vi "imp_test_v8_1.vi"() -> ()   [LabVIEW 2014]
uses:
  <vilib>/LabVIEW Targets/FPGA/cRIO/shared/nicrio_ModuleControls/nicrio_cRIO-9237_DataRatesRing.ctl
  <vilib>/LabVIEW Targets/FPGA/cRIO/shared/nicrio_ModuleControls/nicrio_cRIO-9237_ExcitationVoltageRing.ctl
  <vilib>/rvi/FXPMathLib/FxpSinAndCos/subVIs/nifxpmath_SinAndCos_SimConfig.ctl
  <vilib>/rvi/Emulation/niFpgaGetClockAttributes.vi
  <vilib>/rvi/Emulation/niFpgaSctlEmulationGetInTimedLoop.vi
  <vilib>/rvi/Emulation/niFpgaEmulationReportErrorSimple.vi
  <vilib>/rvi/Emulation/niFpgaProcessEmulError.vi
  <vilib>/rvi/interface/RandomDataEmulation/nirviRandomDataMultiElementFPGAFIFO.vi
  <instcachedir>/0/nirviRandomDataMultiElementFPGAFIFO_AD0CFC12EF974623A9C2E4184BC062B2.lvgen/nirviRandomDataMultiElementFPGAFIFO_AD0CFC12EF974623A9C2E4184BC062B2_025.vi
  <vilib>/rvi/interface/RandomDataEmulation/niFpgaRandomDataHandleErrors.vi
  <vilib>/rvi/Emulation/niFpgaCriticalErrorInLSC.vi
  <vilib>/rvi/FXPMathLib/FxpSinAndCos/simVIs/DllFxpSinAndCosTemp_sub.vi
  <vilib>/rvi/eio/common/nirviEmuTemplateMethod_errors.vi
  <vilib>/rvi/eio/common/nirviEmuTemplatePropertySet_errors.vi
  <vilib>/rvi/DataTransferAndStorage/Container/XNode/niFpgaContainer.xnode
  <vilib>/rvi/interface/RandomDataEmulation/nirviRandomDataFpgaMultiElementTemplate.vi
  <vilib>/rvi/FXPMathLib/FxpSinAndCos/XNode/nifxpmath_SinAndCos.xnode
  <vilib>/eio/EIONode/EIONode.xnode
  <vilib>/rvi/Analysis/measure/butterworth/XNode/niFpgaButterworthFilter.xnode
  <vilib>/eio/EIOPropertyNode/EIOPropertyNode.xnode
  <vilib>/rvi/eio/common/nirviEmuTemplatePropertyGet_errors.vi
  <vilib>/rvi/eio/common/nirviEmuTemplatePropertyGet_noerrors.vi
  <vilib>/rvi/eio/common/nirviEmuTemplatePropertySet_noerrors.vi
panel:
  out "Dy_d (Mavg w. f.)":fxp<+/-,36,14>
  out "Dp_d (Mavg w. f.)":fxp<+/-,36,14>
  in  "Dp_d (Mavg) coeff.":i32[](array[numeric])=[946630756, 63555534]
  in  "Dy_d (Mavg) coeff.":i32[](array[numeric])=[946630756, 63555534]
  out "omega_y (Mavg w. f.)":fxp<+/-,36,14>
  in  "omega_y(Mavg) coeff.":i32[](array[numeric])=[946630756, 63555534]
  out "omega_p (Mavg w. f)":fxp<+/-,36,14>
  in  "omega_P(Mavg) coeff.":i32[](array[numeric])=[946630756, 63555534]
  in  "FIFO":i16(ring) items=["Pitch_F+P", "imp ctrl", "Yaw_F+P"]
  out "PID (kHz)":fxp<+/-,20,10>
  in  "Set 6":bool
  in  "Set 5":bool
  in  "Set 4":bool
  in  "Set 3":bool
  in  "Set 2":bool
  in  "Set 1":bool
  out "Dy1_d (T)":fxp<+/-,36,13>
  out "omega_y1 (T)":fxp<+/-,36,13>
  out "Dp1_d (T)":fxp<+/-,36,13>
  out "omega_p1 (T)":fxp<+/-,36,13>
  out "Dy2_d (T)":fxp<+/-,36,13>
  out "Dp2_d (T)":fxp<+/-,36,13>
  out "omega_y2 (T)":fxp<+/-,36,13>
  out "omega_p2 (T)":fxp<+/-,36,13>
  out "mt_omega_y2":u32
  out "mt_omega_p2":u32
  out "rad_y2":fxp<+/-,33,20>
  out "D_y2":fxp<+/-,32,7>
  out "rad_y1":fxp<+/-,33,20>
  out "D_y1":fxp<+/-,32,7>
  out "Encoder Position_y1":i32
  out "Encoder Position_y2":i32
  out "Encoder Position_p2":i32
  out "D_p2":fxp<+/-,32,7>
  out "rad_p2":fxp<+/-,33,20>
  out "D_p1":fxp<+/-,32,7>
  out "rad_p1":fxp<+/-,33,20>
  out "Encoder Position_p1":i32
  in  "Mag. factor_y":fxp<+/-,20,3>
  in  "Mag. encoder_y":bool
  out "omega_y (rad/s)":fxp<+/-,36,13>
  out "Dy_d (mm/s)":fxp<+/-,36,13>
  in  "Vy. Est.":i16(ring) items=["T", "Mavg", "Mavg w. f."]
  out "omega_y (Mavg)":fxp<+/-,36,14>
  out "Dy_d (Mavg)":fxp<+/-,36,14>
  in  "Dy_d_M_avg_Tc (uSec)":i32
  out "Dp_d (Mavg)":fxp<+/-,36,14>
  out "omega_p (Mavg)":fxp<+/-,36,14>
  in  "Dp_d_M_avg_Tc (uSec)":i32
  out "Dp_d (T)":fxp<+/-,36,13>
  out "omega_p (T)":fxp<+/-,36,13>
  in  "Vp. Est.":i16(ring) items=["T", "Mavg", "Mavg w. f."]
  in  "Mag. factor_p":fxp<+/-,20,3>
  in  "Mag. encoder_p":bool
  in  "Belt_out_p":fxp<+/-,7,7>
  in  "Belt_in_p":fxp<+/-,6,6>
  in  "Belt_out_y":fxp<+/-,7,7>
  in  "Belt_in_y":fxp<+/-,6,6>
  out "Fp_dc":fxp<+/-,32,10>
  out "Fy_dc":fxp<+/-,32,10>
  in  "Zero_y":bool
  in  "Zero_p":bool
  in  "mt0_omega_p":u32
  in  "Encoder reset":bool
  out "fpt_d":fxp<+/-,36,18>
  out "Dp_error_dd":fxp<+/-,36,16>
  out "Dp_error_d":fxp<+/-,33,8>
  in  "Dp_dd coeff.":i32[](array[numeric])=[946630756, 63555534]
  out "Dp_dd":fxp<+/-,36,25>
  out "dFp_PID":fxp<+/-,36,18>
  in  "dFp_PID coeff.":i32[](array[numeric])=[946630756, 63555534]
  out "fpt_i":fxp<+/-,34,18>
  in  "Bv_p":fxp<+/-,22,8>
  in  "Kv_p":fxp<+/-,22,8>
  out "Dp_error":fxp<+/-,22,7>
  out "Dpr_sin":fxp<+/-,22,7>
  in  "Sin offset_p":fxp<+/-,22,7>
  in  "Sin magnitude_p":fxp<+/-,21,6>
  out "Dpr_sin_dd":fxp<+/-,35,20>
  out "Dpr_sin_d":fxp<+/-,33,15>
  out "Sin omega_p":fxp<+/-,34,9>
  in  "Sin wave freq._p (Hz)":fxp<+/-,32,6>
  in  "Dpr_step":fxp<+/-,22,7>
  out "Dpr_for":fxp<+/-,22,7>
  in  "Command_p":i16(ring) items=["Step", "Sine"]
  in  "Ki_p":fxp<+/-,30,9>
  out "Fp_PID":fxp<+/-,36,16>
  in  "fp_tolorance":fxp<+,22,6>
  out "fp_tilde":fxp<+/-,33,10>
  in  "Kd_p":fxp<+/-,30,9>
  in  "Kp_p":fxp<+/-,32,13>
  out "Fr_p":fxp<+/-,32,10>
  in  "S/F coeff_p":fxp<+/-,25,-10>
  in  "S/F coeff_y":fxp<+/-,25,-10>
  out "va_p":fxp<+/-,36,7>
  out "vb_p":fxp<+/-,37,8>
  out "vq_p_F":fxp<+/-,20,5> format="%.57g"
  out "vd_p_F":fxp<+/-,20,5>
  in  "dFp_add":bool
  in  "Stop motor_p":bool
  out "Force_p":fxp<+/-,32,10>
  in  "Strain selection_p":i16(ring) items=["Raw", "Avg.8", "Avg.8 w. filter"]
  out "Strain_p (Avg8 w. f)":fxp<+/-,36,8>
  in  "Strain_p Avg.8 coeff.":i32[](array[numeric])=[946630756, 63555534]
  out "Strain_p (Avg8)":fxp<+/-,36,4>
  out "Raw Strain_p":fxp<+/-,36,4>
  out "Mod6/AI3":fxp<+/-,36,4>
  in  "Strain gage reset_p":bool
  out "Dp_d (mm/s)":fxp<+/-,36,13>
  out "omega_p (rad/s)":fxp<+/-,36,13>
  out "mt_omega_p1":u32
  out "rad_p(NrTheta)":fxp<+/-,33,20>
  out "D_p(mm)":fxp<+/-,32,7>
  out "Encoder Position_p":i32
  in  "Encoder reset_p":bool
  out "Strain_y (Avg8 w. f)":fxp<+/-,36,8>
  in  "Strain_y Avg8 coeff.":i32[](array[numeric])=[-898916953, 1957103773, 3888751]
  out "Dyr_for":fxp<+/-,22,7>
  in  "Command_y":i16(ring) items=["Step", "Sine"]
  out "Strain_y (Avg8)":fxp<+/-,36,4>
  in  "Strain selection_y":i16(ring) items=["Raw", "Avg.8", "Avg.8 w. filter"]
  out "vb_y":fxp<+/-,38,8>
  out "va_y":fxp<+/-,38,8>
  out "fyt_d":fxp<+/-,36,18>
  out "Fr_y":fxp<+/-,32,10>
  in  "Bv_y":fxp<+/-,22,8>
  out "Dy_error_dd":fxp<+/-,36,16>
  out "Dy_error_d":fxp<+/-,33,8>
  in  "Kv_y":fxp<+/-,22,8>
  out "Dy_error":fxp<+/-,22,7>
  out "Dyr_sin_dd":fxp<+/-,35,20>
  out "Dyr_sin_d":fxp<+/-,33,15>
  out "Sin omega_y":fxp<+/-,34,9>
  out "Dyr_sin":fxp<+/-,22,7>
  in  "Sin offset_y":fxp<+/-,22,7>
  in  "Sin magnitude_y":fxp<+/-,21,6>
  out "Time now(s)":fxp<+,52,14>
  in  "Sin wave freq._y (Hz)":fxp<+/-,32,6>
  in  "Dyr_step":fxp<+/-,22,7>
  in  "Drive mode":i16(ring) items=["Backward", "Forward"]
  out "Dy_dd":fxp<+/-,36,25>
  in  "Dy_dd coeff.":i32[](array[numeric])=[946630756, 63555534]
  out "dFy_PID":fxp<+/-,36,18>
  in  "dFy_PID coeff.":i32[](array[numeric])=[946630756, 63555534]
  out "fyt_i":fxp<+/-,36,16>
  out "Fy_PID":fxp<+/-,36,16>
  in  "fy_tolorance":fxp<+,22,6>
  in  "Ki_y":fxp<+/-,30,9>
  in  "Kd_y":fxp<+/-,30,9>
  out "fy_tilde":fxp<+/-,32,10>
  in  "Kp_y":fxp<+/-,32,13>
  out "vq_y_F":fxp<+/-,20,5> format="%.57g"
  out "vd_y_F":fxp<+/-,20,5>
  in  "dFy_add":bool
  in  "Stop motor_y":bool
  out "Dy_d (T)":fxp<+/-,36,13>
  out "omega_y (T)":fxp<+/-,36,13>
  in  "mt0_omega_y":u32
  out "mt_omega_y1":u32
  out "rad_y(NrTheta)":fxp<+/-,33,20>
  out "D_y(mm)":fxp<+/-,32,7>
  out "Encoder Position_y":i32
  in  "Encoder reset_y":bool
  in  "Ini coe.":bool
  out "Loop rate (kHz)":fxp<+/-,36,7>
  out "Force_y":fxp<+/-,32,10>
  out "Raw Strain_y":fxp<+/-,36,4>
  in  "Strain gage reset_y":bool
  in  "Stop (Strain)":bool
  out "Mod6/AI2":fxp<+/-,36,4>
  in  "Excitation Voltage":T1 items=["2.5 Volts", "3.3 Volts", "5.0 Volts", "10.0 Volts", "External Excitation"]
  in  "Data Rate":T2=1 items=["50.000 kS/s (NI 9237)"=1, "25.000 kS/s (NI 9237)"=2, "16.667 kS/s (NI 9237)"=3, "12.500 kS/s (NI 9237)"=4, "10.000 kS/s (NI 9237)"=5, "8.333 kS/s (NI 9237)"=6, "7.143 kS/s (NI 9237)"=7, "6.250 kS/s (NI 9237)"=8, "5.556 kS/s (NI 9237)"=9, "5.000 kS/s (NI 9237)"=10, "4.545 kS/s (NI 9237)"=11, "4.167 kS/s (NI 9237)"=12, "3.846 kS/s (NI 9237)"=13, "3.571 kS/s (NI 9237)"=14, "3.333 kS/s (NI 9237)"=15, "3.125 kS/s (NI 9237)"=16, "2.941 kS/s (NI 9237)"=17, "2.778 kS/s (NI 9237)"=18, "2.632 kS/s (NI 9237)"=19, "2.500 kS/s (NI 9237)"=20, "2.381 kS/s (NI 9237)"=21, "2.273 kS/s (NI 9237)"=22, "2.174 kS/s (NI 9237)"=23, "2.083 kS/s (NI 9237)"=24, "2.000 kS/s (NI 9237)"=25, "1.923 kS/s (NI 9237)"=26, "1.852 kS/s (NI 9237)"=27, "1.786 kS/s (NI 9237)"=28, "1.724 kS/s (NI 9237)"=29, "1.667 kS/s (NI 9237)"=30, "1.613 kS/s (NI 9237)"=31]
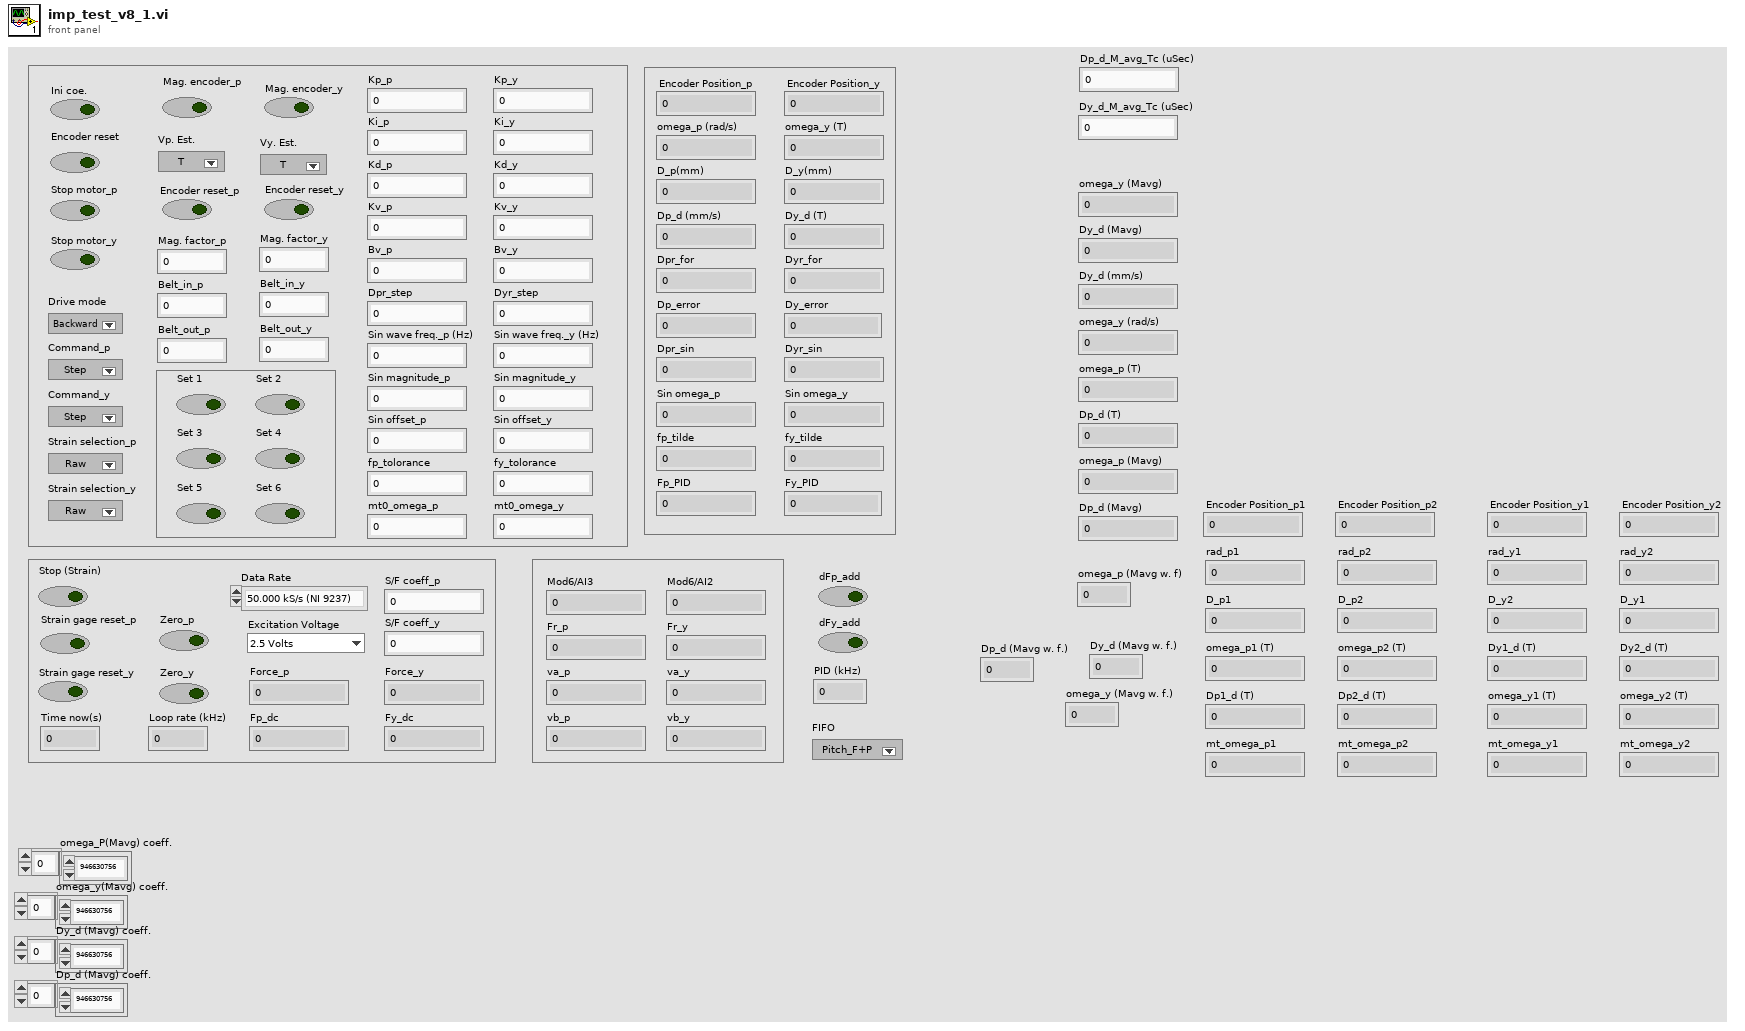
[diagram p1: front panel]
types:
  T1 = typedef "nicrio_cRIO-9237_ExcitationVoltageRing.ctl" = u8
  T2 = typedef "nicrio_cRIO-9237_DataRatesRing.ctl" = u8
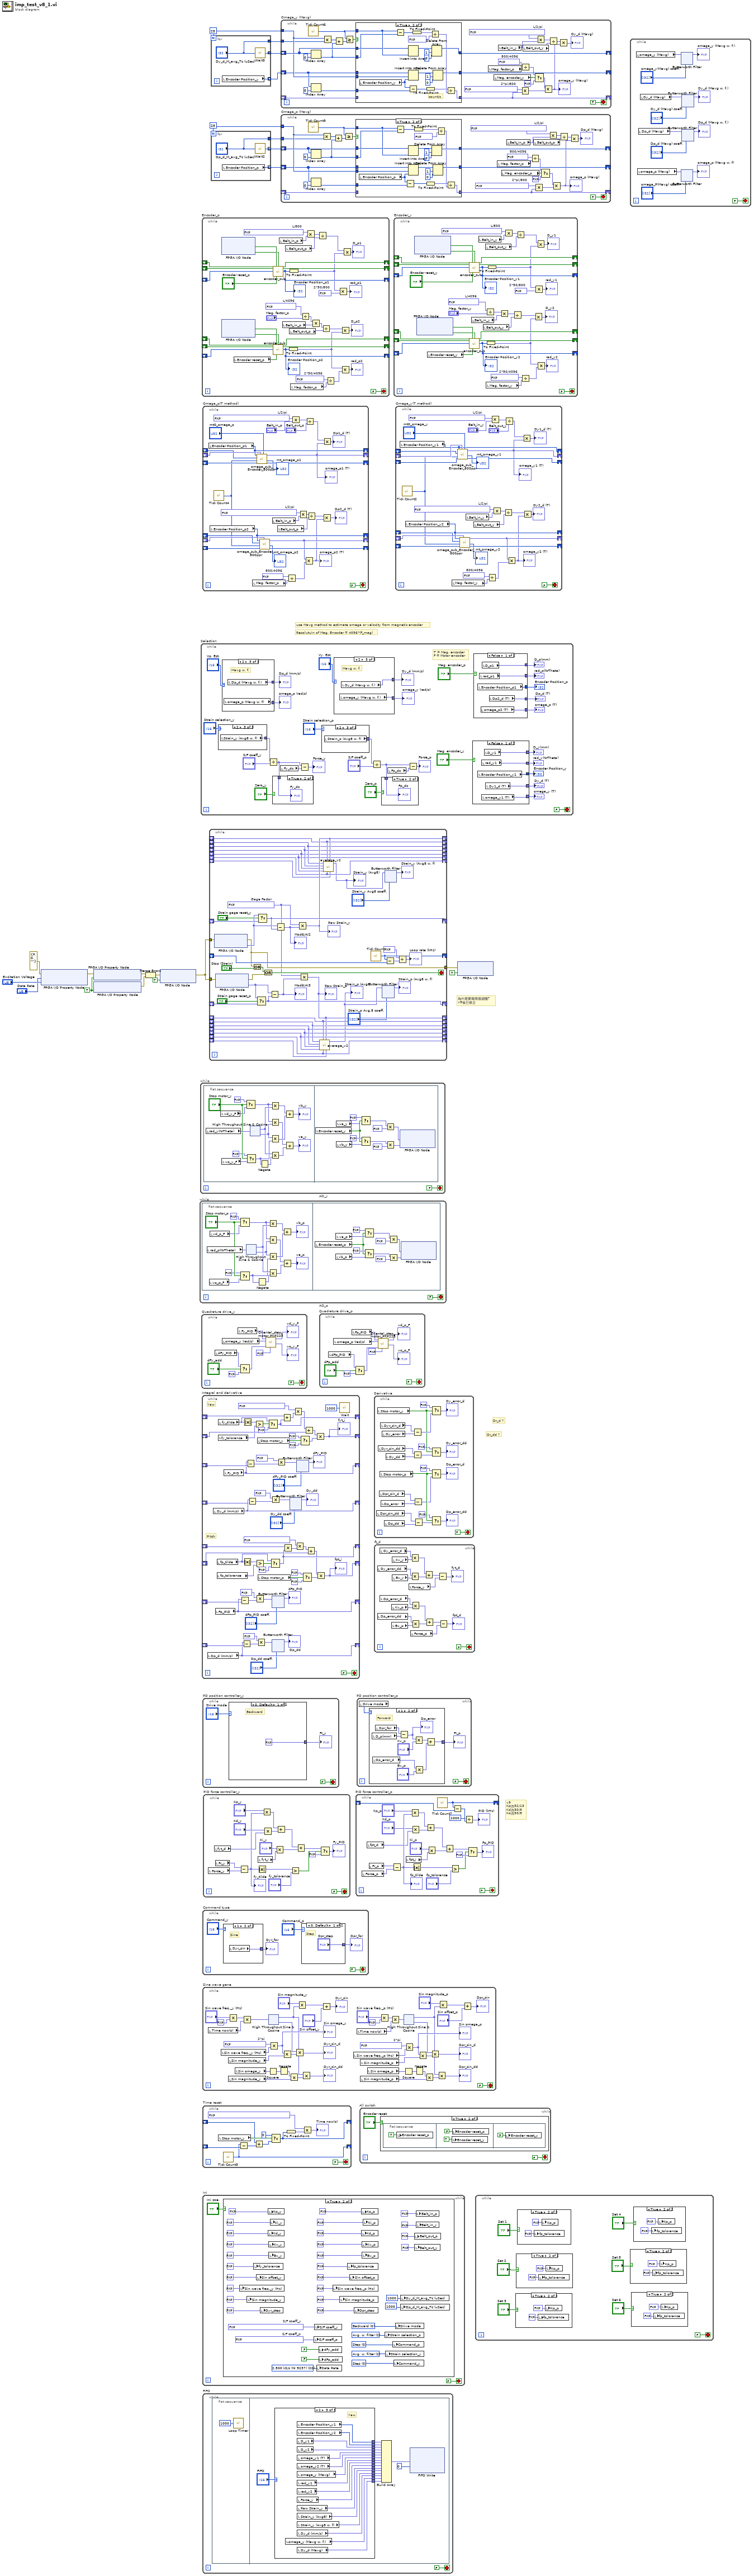
[diagram p0: block diagram]
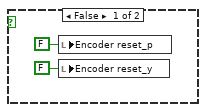
[diagram p10: hidden frame]
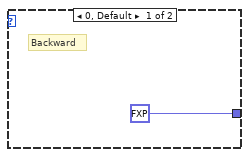
[diagram p11: hidden frame]
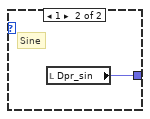
[diagram p12: hidden frame]
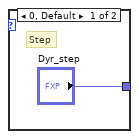
[diagram p13: hidden frame]
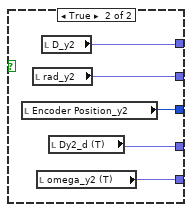
[diagram p14: hidden frame]
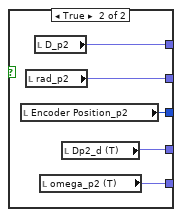
[diagram p15: hidden frame]
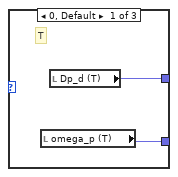
[diagram p16: hidden frame]
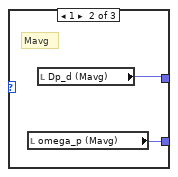
[diagram p17: hidden frame]
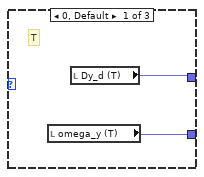
[diagram p18: hidden frame]
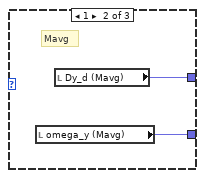
[diagram p19: hidden frame]
diagram:
  w5 = 25
  w8 = 25
  w13 = TRUE ("Half-Bridge Enable")
  # "v9\nKp改32/13\nKd改30/9\nKo改30/9"
  # "Resolutuin of Mag. Encoder = 4096*(F_mag)"
  # "use Mavg method to estimate omega or velocity from magnetic encoder"
  # "為什麼要寫兩個迴圈?\nv9後已修正"
  # "Dr_dd ?"
  # "Dr_d ?"
  n1 = xnode "FPGA I/O Property Node"("error in"=errorcluster {"status"=FALSE, "code"=0, "source"=""}, "Data Rate"="Data Rate", "Excitation Voltage"="Excitation Voltage") -> ("error out"=w18:errorcluster)  [unwired: 1 in, 1 out]
  n2 = xnode "FPGA I/O Property Node"("error in"=w18, "Half-Bridge Enable"=w13) -> ("error out"=w11:errorcluster)  [unwired: 1 in, 1 out]
  n3 = xnode "FPGA I/O Property Node"("Half-Bridge Enable"=w13) -> ("error out"=w10:errorcluster)  [unwired: 2 in, 1 out]
  n4 = Merge Errors(w11, w10) -> (w12:errorcluster)
  n5 = xnode "FPGA I/O Node"("error in"=w12, "Mod6/Start"=TRUE) -> ("error out"=w16:errorcluster)  [unwired: 1 in, 1 out]
  n6 = while "AO_p" {
    stop <- FALSE stop-if-true
    n7 = flat-sequence {
      frame #0 {
        n8 = local read "rad_p(NrTheta)"() -> (w33:fxp<+/-,33,20>)
        n9 = local read "vq_p_F"() -> (w34:fxp<+/-,20,5>)
        n10 = local read "vd_p_F"() -> (w36:fxp<+/-,20,5>)
        n11 = Select(t=fxp<+/-,20,5> 0.0, s="Stop motor_p", f=w36) -> (s? t:f=w25:fxp<+/-,20,5>)
        n12 = Select(t=fxp<+,1,1> 0.0, s="Stop motor_p", f=w34) -> (s? t:f=w24:fxp<+/-,20,5>)
        n13 = xnode "High Throughput Sine & Cosine"("x (pi)"=w33) -> ("sin(x)"=w27:fxp<+/-,16,2>, "cos(x)"=w26:fxp<+/-,16,2>)
        n14 = Negate(x=w24) -> (-x=w32:fxp<+/-,21,6>)
        n15 = Multiply(x=w25, y=w27) -> (x*y=w31:fxp<+/-,36,7>)
        n16 = Multiply(x=w25, y=w26) -> (x*y=w29:fxp<+/-,36,7>)
        n17 = Multiply(x=w26, y=w24) -> (x*y=w30:fxp<+/-,36,7>)
        n18 = Multiply(x=w27, y=w32) -> (x*y=w28:fxp<+/-,35,6>)
        n19 = Add(x=w31, y=w30) -> (x+y=→"vb_p":fxp<+/-,37,8>)
        n20 = Add(x=w29, y=w28) -> (x+y=→"va_p":fxp<+/-,36,7>)
      }
      frame #1 {
        n21 = local read "Encoder reset_p"() -> (w69:bool)
        n22 = local read "vb_p"() -> (w70:fxp<+/-,37,8>)
        n23 = local read "va_p"() -> (w71:fxp<+/-,36,7>)
        n24 = Select(t=fxp<+,2,2> 3.0, s=w69, f=w71) -> (s? t:f=w77:fxp<+/-,36,7>)
        n25 = Select(t=fxp<+,1,1> 0.0, s=w69, f=w70) -> (s? t:f=w76:fxp<+/-,37,8>)
        n26 = Multiply(x=w77, y=fxp<+/-,1,0> -0.5) -> (x*y=w72:fxp<+/-,36,6>)
        n27 = Multiply(x=w76, y=fxp<+/-,1,0> -0.5) -> (x*y=w73:fxp<+/-,36,6>)
        n28 = xnode "FPGA I/O Node"("Mod8/AO0"=w72, "Mod8/AO1"=w73) -> ()  [unwired: 2 in, 2 out]
      }
    }
  }
  n29 = while "AO_y" {
    stop <- FALSE stop-if-true
    n30 = flat-sequence {
      frame #0 {
        n31 = local read "rad_y(NrTheta)"() -> (w97:fxp<+/-,33,20>)
        n32 = local read "vd_y_F"() -> (w95:fxp<+/-,20,5>)
        n33 = local read "vq_y_F"() -> (w94:fxp<+/-,20,5>)
        n34 = Select(t=fxp<+/-,20,5> 0.0, s="Stop motor_y", f=w95) -> (s? t:f=w89:fxp<+/-,20,5>)
        n35 = Select(t=fxp<+/-,20,5> 0.0, s="Stop motor_y", f=w94) -> (s? t:f=w88:fxp<+/-,20,5>)
        n36 = xnode "High Throughput Sine & Cosine"("x (pi)"=w97) -> ("sin(x)"=w91:fxp<+/-,17,2>, "cos(x)"=w90:fxp<+/-,17,2>)
        n37 = Negate(x=w88) -> (-x=w87:fxp<+/-,21,6>)
        n38 = Multiply(x=w89, y=w91) -> (x*y=w86:fxp<+/-,37,7>)
        n39 = Multiply(x=w89, y=w90) -> (x*y=w84:fxp<+/-,37,7>)
        n40 = Multiply(x=w90, y=w88) -> (x*y=w85:fxp<+/-,37,7>)
        n41 = Multiply(x=w91, y=w87) -> (x*y=w83:fxp<+/-,36,6>)
        n42 = Add(x=w86, y=w85) -> (x+y=→"vb_y":fxp<+/-,38,8>)
        n43 = Add(x=w84, y=w83) -> (x+y=→"va_y":fxp<+/-,37,7>)
      }
      frame #1 {
        n44 = local read "Encoder reset_y"() -> (w130:bool)
        n45 = local read "va_y"() -> (w129:fxp<+/-,38,8>)
        n46 = local read "vb_y"() -> (w128:fxp<+/-,38,8>)
        n47 = Select(t=fxp<+,2,2> 3.0, s=w130, f=w129) -> (s? t:f=w134:fxp<+/-,38,8>)
        n48 = Select(t=fxp<+,1,1> 0.0, s=w130, f=w128) -> (s? t:f=w133:fxp<+/-,38,8>)
        n49 = Multiply(x=w134, y=fxp<+/-,1,0> -0.5) -> (x*y=w137:fxp<+/-,39,8>)
        n50 = Multiply(x=w133, y=fxp<+/-,1,0> -0.5) -> (x*y=w138:fxp<+/-,37,6>)
        n51 = xnode "FPGA I/O Node"("Mod8/AO2"=w137, "Mod8/AO3"=w138) -> ()  [unwired: 2 in, 2 out]
      }
    }
  }
  n52 = while "Selection" {
    stop <- FALSE stop-if-true
    # "T = Mag. encoder\nF = Motor encoder"
    n53 = case shown="2" "Strain selection_y" {
      tunnel: [w209 w210 w211] -> w170
      frame 0, Default {
        n54 = local read "Raw Strain_y"() -> (w209:fxp<+/-,36,4>)
      }
      frame 1 {
        n55 = local read "Strain_y (Avg8)"() -> (w210:fxp<+/-,36,4>)
      }
      frame 2 {
        n56 = local read "Strain_y (Avg8 w. f)"() -> (w211:fxp<+/-,36,8>)
      }
    }
    n57 = case shown="2" "Vp. Est." {
      tunnel: [w193 w194 w197] -> w153
      tunnel: [w192 w195 w196] -> w154
      frame 0, Default {
        # "T"
        n58 = local read "omega_p (T)"() -> (w193:fxp<+/-,36,13>)
        n59 = local read "Dp_d (T)"() -> (w192:fxp<+/-,36,13>)
      }
      frame 1 {
        # "Mavg"
        n60 = local read "omega_p (Mavg)"() -> (w194:fxp<+/-,36,14>)
        n61 = local read "Dp_d (Mavg)"() -> (w195:fxp<+/-,36,14>)
      }
      frame 2 {
        # "Mavg w. f."
        n62 = local read "omega_p (Mavg w. f)"() -> (w197:fxp<+/-,36,14>)
        n63 = local read "Dp_d (Mavg w. f.)"() -> (w196:fxp<+/-,36,14>)
      }
    }
    "Dp_d (mm/s)" <- w154
    "omega_p (rad/s)" <- w153
    n64 = Divide(x=w170, y="S/F coeff_y") -> (x/y=w163:fxp<+/-,32,10>)
    n65 = case shown="True" "Zero_y" {
      tunnel: w163 -> [_ w205]
      frame False {
      }
      frame True {
        "Fy_dc" <- w205
      }
    }
    n66 = local read "Fy_dc"() -> (w164:fxp<+/-,32,10>)
    n67 = Subtract(x=w163, y=w164) -> (x-y=→"Force_y":fxp<+/-,33,11>)
    n68 = case shown="2" "Strain selection_p" {
      tunnel: [w206 w207 w208] -> w168
      frame 0, Default {
        n69 = local read "Raw Strain_p"() -> (w206:fxp<+/-,36,4>)
      }
      frame 1 {
        n70 = local read "Strain_p (Avg8)"() -> (w207:fxp<+/-,36,4>)
      }
      frame 2 {
        n71 = local read "Strain_p (Avg8 w. f)"() -> (w208:fxp<+/-,36,8>)
      }
    }
    n72 = case shown="2" "Vy. Est." {
      tunnel: [w199 w201 w203] -> w156
      tunnel: [w198 w200 w202] -> w157
      frame 0, Default {
        # "T"
        n73 = local read "omega_y (T)"() -> (w198:fxp<+/-,36,13>)
        n74 = local read "Dy_d (T)"() -> (w199:fxp<+/-,36,13>)
      }
      frame 1 {
        # "Mavg"
        n75 = local read "omega_y (Mavg)"() -> (w200:fxp<+/-,36,14>)
        n76 = local read "Dy_d (Mavg)"() -> (w201:fxp<+/-,36,14>)
      }
      frame 2 {
        # "Mavg w. f."
        n77 = local read "omega_y (Mavg w. f.)"() -> (w202:fxp<+/-,36,14>)
        n78 = local read "Dy_d (Mavg w. f.)"() -> (w203:fxp<+/-,36,14>)
      }
    }
    "Dy_d (mm/s)" <- w156
    "omega_y (rad/s)" <- w157
    n79 = Divide(x=w168, y="S/F coeff_p") -> (x/y=w160:fxp<+/-,32,10>)
    n80 = case shown="True" "Zero_p" {
      tunnel: w160 -> [_ w204]
      frame False {
      }
      frame True {
        "Fp_dc" <- w204
      }
    }
    n81 = local read "Fp_dc"() -> (w158:fxp<+/-,32,10>)
    n82 = Subtract(x=w160, y=w158) -> (x-y=→"Force_p":fxp<+/-,33,11>)
    n83 = case shown="False" "Mag. encoder_y" {
      tunnel: [w176 w180] -> w144
      tunnel: [w175 w181] -> w145
      tunnel: [w174 w179] -> w147
      tunnel: [w172 w178] -> w141
      tunnel: [w173 w177] -> w140
      frame False {
        n84 = local read "Encoder Position_y1"() -> (w174:i32)
        n85 = local read "rad_y1"() -> (w176:fxp<+/-,33,20>)
        n86 = local read "omega_y1 (T)"() -> (w172:fxp<+/-,36,13>)
        n87 = local read "D_y1"() -> (w175:fxp<+/-,32,7>)
        n88 = local read "Dy1_d (T)"() -> (w173:fxp<+/-,36,13>)
      }
      frame True {
        n89 = local read "Encoder Position_y2"() -> (w179:i32)
        n90 = local read "rad_y2"() -> (w180:fxp<+/-,33,20>)
        n91 = local read "omega_y2 (T)"() -> (w178:fxp<+/-,36,13>)
        n92 = local read "D_y2"() -> (w181:fxp<+/-,32,7>)
        n93 = local read "Dy2_d (T)"() -> (w177:fxp<+/-,36,13>)
      }
    }
    "D_y(mm)" <- w145
    "rad_y(NrTheta)" <- w144
    "Encoder Position_y" <- w147
    "Dy_d (T)" <- w140
    "omega_y (T)" <- w141
    n94 = case shown="False" "Mag. encoder_p" {
      tunnel: [w186 w191] -> w149
      tunnel: [w185 w190] -> w150
      tunnel: [w184 w189] -> w151
      tunnel: [w182 w188] -> w143
      tunnel: [w183 w187] -> w142
      frame False {
        n95 = local read "Encoder Position_p1"() -> (w184:i32)
        n96 = local read "rad_p1"() -> (w185:fxp<+/-,33,20>)
        n97 = local read "omega_p2 (T)"() -> (w182:fxp<+/-,36,13>)
        n98 = local read "D_p1"() -> (w186:fxp<+/-,32,7>)
        n99 = local read "Dp2_d (T)"() -> (w183:fxp<+/-,36,13>)
      }
      frame True {
        n100 = local read "Encoder Position_p2"() -> (w189:i32)
        n101 = local read "rad_p2"() -> (w190:fxp<+/-,33,20>)
        n102 = local read "D_p2"() -> (w191:fxp<+/-,32,7>)
        n103 = local read "omega_p2 (T)"() -> (w188:fxp<+/-,36,13>)
        n104 = local read "Dp2_d (T)"() -> (w187:fxp<+/-,36,13>)
      }
    }
    "D_p(mm)" <- w149
    "rad_p(NrTheta)" <- w150
    "Encoder Position_p" <- w151
    "Dp_d (T)" <- w142
    "omega_p (T)" <- w143
  }
  n105 = while "Quadrature drive_y" {
    stop <- FALSE stop-if-true
    n106 = local read "dFy_PID"() -> (w213:fxp<+/-,36,18>)
    n107 = local read "omega_y (rad/s)"() -> (w221:fxp<+/-,36,13>)
    n108 = local read "Fy_PID"() -> (w214:fxp<+/-,36,16>)
    n109 = Select(t=w213, s="dFy_add", f=fxp<+,1,1> 0.0) -> (s? t:f=w217:fxp<+/-,36,18>)
    n110 = call "Oriental_step_motor_PKP225.vi"("F_Threshold"=fxp<+,12,12> 10.0, "dFmr"=w217, "omega"=w221, "Fmr"=w214) -> ("vq_F"=→"vq_y_F":fxp<+/-,20,5>, "vd_F"=→"vd_y_F":fxp<+/-,20,5>)  [unwired: 6 in]
  }
  n111 = while "Encoder_p" {
    shift-right: [w259] -> _
    shift-left: _ -> [w258]
    shift-right: [w260] -> _
    shift-left: _ -> [w257]
    shift-right: [w254] -> _
    shift-left: _ -> [w256]
    shift-right: [w245] -> _
    shift-left: _ -> [w244]
    shift-right: [w246] -> _
    shift-left: _ -> [w247]
    shift-right: [w241] -> _
    shift-left: _ -> [w242]
    stop <- FALSE stop-if-true
    w237 = fxp<+/-,20,-5> 0.00048828125  # L/4096
    w235 = fxp<+/-,16,1> 0.0244140625  # 2*50/4096
    w253 = fxp<+/-,20,-5> 0.002499997615814209  # L/800
    w227 = fxp<+/-,16,1> 0.125  # 2*50/800
    n112 = xnode "FPGA I/O Node"() -> ("Mod4/DI0"=w262:bool, "Mod4/DI1"=w261:bool)  [unwired: 2 in, 2 out]
    n113 = xnode "FPGA I/O Node"() -> ("Mod4/DI3"=w249:bool, "Mod4/DI4"=w248:bool)  [unwired: 2 in, 2 out]
    n114 = local read "Encoder reset_p"() -> (w243:bool)
    n115 = call "encoder_sub.vi"("A_pre"=w258, "B_pre"=w257, "Encoder Position_pre"=w256, "A input"=w262, "Encoder Position Reset"="Encoder reset_p", "B input"=w261) -> ("A"=w259:bool, "B"=w260:bool, "Encoder Position (Counts)"=w254:i32)  [unwired: 19 in]
    "Encoder Position_p1" <- w254
    n116 = call "encoder_sub.vi"("A_pre"=w244, "B_pre"=w247, "Encoder Position_pre"=w242, "A input"=w249, "Encoder Position Reset"=w243, "B input"=w248) -> ("A"=w245:bool, "B"=w246:bool, "Encoder Position (Counts)"=w241:i32)  [unwired: 19 in]
    "Encoder Position_p2" <- w241
    n117 = local read "Belt_in_p"() -> (w252:fxp<+/-,6,6>)
    n118 = local read "Belt_in_p"() -> (w238:fxp<+/-,6,6>)
    n119 = local read "Belt_out_p"() -> (w250:fxp<+/-,7,7>)
    n120 = To Fixed-Point(number=w241) -> (fixed-point=w223:fxp<+/-,32,32>)  [unwired: 1 in]
    n121 = To Fixed-Point(number=w254) -> (fixed-point=w228:fxp<+/-,32,32>)  [unwired: 1 in]
    n122 = local read "Belt_out_p"() -> (w240:fxp<+/-,7,7>)
    n123 = local read "Mag. factor_p"() -> (w234:fxp<+/-,20,3>)
    n124 = Divide(x=w237, y="Mag. factor_p") -> (x/y=w236:fxp<+/-,41,13>)
    n125 = Multiply(x=w253, y=w252) -> (x*y=w251:fxp<+/-,26,1>)
    n126 = Multiply(x=w236, y=w238) -> (x*y=w239:fxp<+/-,46,18>)
    n127 = Divide(x=w251, y=w250) -> (x/y=w230:fxp<+/-,33,1>)
    n128 = Divide(x=w239, y=w240) -> (x/y=w225:fxp<+/-,53,18>)
    n129 = Divide(x=w235, y=w234) -> (x/y=w222:fxp<+/-,32,1>)
    n130 = Multiply(x=w228, y=w227) -> (x*y=→"rad_p1":fxp<+/-,33,20>)
    n131 = Multiply(x=w225, y=w223) -> (x*y=→"D_p2":fxp<+/-,37,7>)
    n132 = Multiply(x=w223, y=w222) -> (x*y=→"rad_p2":fxp<+/-,33,20>)
    n133 = Multiply(x=w230, y=w228) -> (x*y=→"D_p1":fxp<+/-,32,7>)
  }
  n134 = while "Integral and derivative" {
    shift-right: [w318] -> _
    shift-left: _ -> [w317]
    shift-right: [w310] -> _
    shift-left: _ -> [w309]
    shift-right: [w320] -> _
    shift-left: _ -> [w321]
    shift-right: [w300] -> _
    shift-left: _ -> [w299]
    shift-right: [w286] -> _
    shift-left: _ -> [w289]
    shift-right: [w279] -> _
    shift-left: _ -> [w278]
    shift-right: [w273] -> _
    shift-left: _ -> [w272]
    shift-right: [w268] -> _
    shift-left: _ -> [w269]
    stop <- FALSE stop-if-true
    # "Pitch"
    # "Yaw"
    n135 = local read "Dp_d (mm/s)"() -> (w268:fxp<+/-,36,13>)
    n136 = local read "Dy_d (mm/s)"() -> (w300:fxp<+/-,36,13>)
    n137 = local read "Fp_PID"() -> (w273:fxp<+/-,36,16>)
    n138 = local read "fp_tilde"() -> (w290:fxp<+/-,33,10>)
    n139 = local read "fp_tolorance"() -> (w293:fxp<+,22,6>)
    n140 = local read "fy_tolorance"() -> (w296:fxp<+,22,6>)
    n141 = local read "fy_tilde"() -> (w322:fxp<+/-,32,10>)
    n142 = local read "Fy_PID"() -> (w320:fxp<+/-,36,16>)
    n143 = Subtract(x=w273, y=w272) -> (x-y=w277:fxp<+/-,37,17>)
    n144 = Subtract(x=w268, y=w269) -> (x-y=w270:fxp<+/-,37,14>)
    n145 = Absolute Value(x=w290) -> (abs(x)=w294:fxp<+,33,10>)
    n146 = Absolute Value(x=w322) -> (abs(x)=w324:fxp<+,32,10>)
    n147 = Subtract(x=w320, y=w321) -> (x-y=w308:fxp<+/-,37,17>)
    n148 = Subtract(x=w300, y=w299) -> (x-y=w302:fxp<+/-,36,11>)
    n149 = Greater?(x=w324, y=w296) -> (0:w325:bool)
    n150 = Greater?(x=w294, y=w293) -> (0:w292:bool)
    n151 = Multiply(x=fxp<+,7,10> 1000.0, y=w277) -> (x*y=w275:fxp<+/-,32,18>)
    n152 = Multiply(x=fxp<+,7,10> 1000.0, y=w270) -> (x*y=w266:fxp<+/-,36,21>)
    n153 = local read "Stop motor_y"() -> (w311:bool)
    n154 = local read "Stop motor_p"() -> (w281:bool)
    n155 = Select(t=w322, s=w325, f=fxp<+/-,33,11> 0.0) -> (s? t:f=w318:fxp<+/-,33,11>)
    n156 = Select(t=w290, s=w292, f=fxp<+,1,1> 0.0) -> (s? t:f=w286:fxp<+/-,33,10>)
    n157 = Multiply(x=fxp<+,7,10> 1000.0, y=w302) -> (x*y=w301:fxp<+/-,36,21>)
    n158 = xnode "Butterworth Filter"("input data"=w275, "scaled coefficients"="dFp_PID coeff.") -> ("output data"=→"dFp_PID":fxp<+/-,36,22>)  [unwired: 1 in]
    n159 = xnode "Butterworth Filter"("input data"=w266, "scaled coefficients"="Dp_dd coeff.") -> ("output data"=→"Dp_dd":fxp<+/-,36,25>)  [unwired: 1 in]
    n160 = Multiply(x=fxp<+,7,10> 1000.0, y=w308) -> (x*y=w305:fxp<+/-,32,18>)
    n161 = Add(x=w317, y=w318) -> (x+y=w323:fxp<+/-,34,12>)
    n162 = Multiply(x=w289, y=w286) -> (x*y=w288:fxp<+/-,34,12>)
    n163 = xnode "Butterworth Filter"("input data"=w301, "scaled coefficients"="Dy_dd coeff.") -> ("output data"=→"Dy_dd":fxp<+/-,36,25>)  [unwired: 1 in]
    n164 = Multiply(x=fxp<+/-,30,12> 0.000499725341796875, y=w323) -> (x*y=w316:fxp<+/-,34,10>)
    n165 = Multiply(x=fxp<+/-,30,12> 0.000499725341796875, y=w288) -> (x*y=w285:fxp<+/-,34,10>)
    n166 = xnode "Butterworth Filter"("input data"=w305, "scaled coefficients"="dFy_PID coeff.") -> ("output data"=→"dFy_PID":fxp<+/-,36,22>)  [unwired: 1 in]
    n167 = Select(t=fxp<+,1,1> 0.0, s=w311, f=fxp<+,1,1> 1.0) -> (s? t:f=w314:fxp<+,1,1>)
    n168 = Select(t=fxp<+,1,1> 0.0, s=w281, f=fxp<+,1,1> 1.0) -> (s? t:f=w283:fxp<+,1,1>)
    n169 = Add(x=w316, y=w309) -> (x+y=w315:fxp<+/-,36,16>)
    n170 = Add(x=w285, y=w278) -> (x+y=w284:fxp<+/-,36,16>)
    n171 = Multiply(x=w315, y=w314) -> (x*y=w310:fxp<+/-,34,18>)
    "fyt_i" <- w310
    n172 = Multiply(x=w284, y=w283) -> (x*y=w279:fxp<+/-,34,18>)
    "fpt_i" <- w279
    n173 = call "Wait"("Count(uSec)"=u32 1000) -> ()  [unwired: 1 out]
  }
  n174 = while "Omega_p(T method)" {
    shift-right: [w391] -> _
    shift-left: _ -> [w389]
    shift-right: [w362] -> _
    shift-left: _ -> [w390]
    shift-right: [w387] -> _
    shift-left: _ -> [w388]
    shift-right: [w378] -> _
    shift-left: _ -> [w377]
    shift-right: [w371] -> _
    shift-left: _ -> [w376]
    shift-right: [w375] -> _
    shift-left: _ -> [w374]
    stop <- FALSE stop-if-true
    w369 = fxp<+/-,32,0> 0.3183098859153688  # L/2/pi
    w380 = fxp<+,32,0> 0.1953125  # 800/4096
    w384 = fxp<+/-,32,0> 0.3183098859153688  # L/2/pi
    n175 = local read "Encoder Position_p1"() -> (w391:i32)
    n176 = local read "Encoder Position_p2"() -> (w378:i32)
    n177 = call "Tick Count4"() -> ("Tick Count(Ticks)"=w373:u32)
    n178 = local read "Mag. factor_p"() -> (w379:fxp<+/-,20,3>)
    n179 = call "omega_sub_Encoder_800ppr.vi"("mt0"="mt0_omega_p", "omega_pre"=w390, "ticks_m_pre"=w388, "ticks"=w373, "count_pre"=w389, "count"=w391) -> ("ticks_m"=w387:u32, "mt"=→"mt_omega_p1":u32, "omega"=w362:fxp<+/-,36,13>)  [unwired: 3 in]
    "omega_p1 (T)" <- w362
    n180 = call "omega_sub_Encoder_800ppr.vi"("omega_pre"=w376, "ticks_m_pre"=w374, "ticks"=w373, "count_pre"=w377, "count"=w378) -> ("ticks_m"=w375:u32, "mt"=→"mt_omega_p2":u32, "omega"=w371:fxp<+/-,36,13>)  [unwired: 4 in]
    n181 = local read "Belt_in_p"() -> (w367:fxp<+/-,6,6>)
    n182 = local read "Belt_out_p"() -> (w366:fxp<+/-,7,7>)
    n183 = Divide(x=w380, y=w379) -> (x/y=w370:fxp<+/-,32,1>)
    n184 = Multiply(x=w384, y="Belt_in_p") -> (x*y=w382:fxp<+/-,38,6>)
    n185 = Multiply(x=w369, y=w367) -> (x*y=w368:fxp<+/-,38,6>)
    n186 = Multiply(x=w371, y=w370) -> (x*y=w360:fxp<+/-,36,13>)
    "omega_p2 (T)" <- w360
    n187 = Divide(x=w382, y="Belt_out_p") -> (x/y=w363:fxp<+/-,20,1>)
    n188 = Divide(x=w368, y=w366) -> (x/y=w361:fxp<+/-,45,6>)
    n189 = Multiply(x=w361, y=w360) -> (x*y=→"Dp2_d (T)":fxp<+/-,36,13>)
    n190 = Multiply(x=w363, y=w362) -> (x*y=→"Dp1_d (T)":fxp<+/-,36,13>)
  }
  n191 = while "PD position controller_y" {
    stop <- FALSE stop-if-true
    n192 = case shown="0, Default" "Drive mode" {
      tunnel: [fxp<+/-,62,19> 0.0 w397] -> w393
      frame 0, Default {
        # "Backward"
      }
      frame 1 {
        # "Forward"
        n193 = local read "Dy_error_d"() -> (w399:fxp<+/-,33,8>)
        n194 = local read "D_y(mm)"() -> (w404:fxp<+/-,32,7>)
        n195 = local read "Dyr_for"() -> (w396:fxp<+/-,22,7>)
        n196 = Subtract(x=w396, y=w404) -> (x-y=w403:fxp<+/-,33,8>)
        "Dy_error" <- w403
        n197 = Multiply(x=w403, y="Kv_y") -> (x*y=w401:fxp<+/-,54,15>)
        n198 = Multiply(x=w399, y="Bv_y") -> (x*y=w398:fxp<+/-,55,16>)
        n199 = Add(x=w401, y=w398) -> (x+y=w397:fxp<+/-,55,16>)
      }
    }
    "Fr_y" <- w393
  }
  n200 = while "Command type" {
    stop <- FALSE stop-if-true
    n201 = case shown="1" "Command_y" {
      tunnel: ["Dyr_step" w413] -> w408
      frame 0, Default {
        # "Step"
      }
      frame 1 {
        # "Sine"
        n202 = local read "Dyr_sin"() -> (w413:fxp<+/-,22,7>)
      }
    }
    "Dyr_for" <- w408
    n203 = case shown="0, Default" "Command_p" {
      tunnel: ["Dpr_step" w411] -> w406
      frame 0, Default {
        # "Step"
      }
      frame 1 {
        # "Sine"
        n204 = local read "Dpr_sin"() -> (w411:fxp<+/-,22,7>)
      }
    }
    "Dpr_for" <- w406
  }
  n205 = while "Sine wave gene" {
    stop <- FALSE stop-if-true
    w419 = fxp<+,20,3> 6.2831878662109375  # 2*pi
    w451 = fxp<+,20,3> 6.2831878662109375  # 2*pi
    n206 = local read "Time now(s)"() -> (w457:fxp<+,52,14>)
    n207 = local read "Sin wave freq._y (Hz)"() -> (w450:fxp<+/-,32,6>)
    n208 = Multiply(x="Sin wave freq._y (Hz)", y=fxp<+/-,10,3> 2.0) -> (x*y=w458:fxp<+/-,41,9>)
    n209 = local read "Sin magnitude_y"() -> (w448:fxp<+/-,21,6>)
    n210 = local read "Sin magnitude_y"() -> (w441:fxp<+/-,21,6>)
    n211 = local read "Sin omega_y"() -> (w444:fxp<+/-,34,9>)
    n212 = Multiply(x=w458, y=w457) -> (x*y=w456:fxp<+/-,41,19>)
    n213 = Square(x=w444) -> (x^2=w443:fxp<+,34,18>)
    n214 = xnode "High Throughput Sine & Cosine"("x (pi)"=w456) -> ("sin(x)"=w438:fxp<+/-,16,2>, "cos(x)"=w446:fxp<+/-,16,2>)
    n215 = Multiply(x=w451, y=w450) -> (x*y=w449:fxp<+/-,34,9>)
    "Sin omega_y" <- w449
    n216 = Negate(x=w443) -> (-x=w442:fxp<+/-,35,19>)
    n217 = Multiply(x=w449, y=w448) -> (x*y=w447:fxp<+/-,33,15>)
    n218 = Multiply(x=w442, y=w441) -> (x*y=w440:fxp<+/-,34,20>)
    n219 = Multiply(x=w446, y=w447) -> (x*y=→"Dyr_sin_d":fxp<+/-,33,15>)
    n220 = Multiply(x="Sin magnitude_y", y=w438) -> (x*y=w454:fxp<+/-,37,8>)
    n221 = Multiply(x=w438, y=w440) -> (x*y=→"Dyr_sin_dd":fxp<+/-,35,20>)
    n222 = Add(x=w454, y="Sin offset_y") -> (x+y=→"Dyr_sin":fxp<+/-,37,8>)
    n223 = local read "Sin wave freq._p (Hz)"() -> (w415:fxp<+/-,32,6>)
    n224 = local read "Time now(s)"() -> (w433:fxp<+,52,14>)
    n225 = local read "Sin magnitude_p"() -> (w416:fxp<+/-,21,6>)
    n226 = local read "Sin magnitude_p"() -> (w418:fxp<+/-,21,6>)
    n227 = local read "Sin omega_p"() -> (w417:fxp<+/-,34,9>)
    n228 = Multiply(x="Sin wave freq._p (Hz)", y=fxp<+/-,10,3> 2.0) -> (x*y=w437:fxp<+/-,42,9>)
    n229 = Multiply(x=w437, y=w433) -> (x*y=w434:fxp<+/-,41,19>)
    n230 = Square(x=w417) -> (x^2=w429:fxp<+,34,18>)
    n231 = xnode "High Throughput Sine & Cosine"("x (pi)"=w434) -> ("sin(x)"=w420:fxp<+/-,16,2>, "cos(x)"=w425:fxp<+/-,16,2>)
    n232 = Multiply(x=w419, y=w415) -> (x*y=w432:fxp<+/-,34,9>)
    "Sin omega_p" <- w432
    n233 = Negate(x=w429) -> (-x=w428:fxp<+/-,35,19>)
    n234 = Multiply(x=w432, y=w416) -> (x*y=w431:fxp<+/-,33,15>)
    n235 = Multiply(x=w428, y=w418) -> (x*y=w427:fxp<+/-,35,19>)
    n236 = Multiply(x=w425, y=w431) -> (x*y=→"Dpr_sin_d":fxp<+/-,33,15>)
    n237 = Multiply(x=w420, y=w427) -> (x*y=→"Dpr_sin_dd":fxp<+/-,35,20>)
    n238 = Multiply(x="Sin magnitude_p", y=w420) -> (x*y=w423:fxp<+/-,37,8>)
    n239 = Add(x=w423, y="Sin offset_p") -> (x+y=→"Dpr_sin":fxp<+/-,37,8>)
  }
  n240 = while "Time reset" {
    shift-right: [w530] -> _
    shift-left: _ -> [w531]
    shift-right: [w525] -> _
    shift-left: _ -> [w526]
    stop <- FALSE stop-if-true
    n241 = local read "Stop motor_y"() -> (w532:bool)
    n242 = call "Tick Count3"() -> ("Tick Count(uSec)"=w530:u32)
    n243 = Subtract(x=w530, y=w531) -> (x-y=w529:u32)
    n244 = Add(x=w526, y=w529) -> (x+y=w528:u32)
    n245 = Select(t=u32 0, s=w532, f=w528) -> (s? t:f=w525:u32)
    n246 = To Fixed-Point(number=w525) -> (fixed-point=w524:fxp<+,32,32>)  [unwired: 1 in]
    n247 = Multiply(x=fxp<+,20,-18> 1.0000003385357559e-06, y=w524) -> (x*y=→"Time now(s)":fxp<+,52,14>)
  }
  n248 = while "Ini" {
    stop <- FALSE stop-if-true
    n249 = case shown="True" "Ini coe." {
      frame False {
      }
      frame True {
        w536 = T2 20 items=["50.000 kS/s (NI 9237)"=1, "25.000 kS/s (NI 9237)"=2, "16.667 kS/s (NI 9237)"=3, "12.500 kS/s (NI 9237)"=4, "10.000 kS/s (NI 9237)"=5, "8.333 kS/s (NI 9237)"=6, "7.143 kS/s (NI 9237)"=7, "6.250 kS/s (NI 9237)"=8, "5.556 kS/s (NI 9237)"=9, "5.000 kS/s (NI 9237)"=10, "4.545 kS/s (NI 9237)"=11, "4.167 kS/s (NI 9237)"=12, "3.846 kS/s (NI 9237)"=13, "3.571 kS/s (NI 9237)"=14, "3.333 kS/s (NI 9237)"=15, "3.125 kS/s (NI 9237)"=16, "2.941 kS/s (NI 9237)"=17, "2.778 kS/s (NI 9237)"=18, "2.632 kS/s (NI 9237)"=19, "2.500 kS/s (NI 9237)"=20, "2.381 kS/s (NI 9237)"=21, "2.273 kS/s (NI 9237)"=22, "2.174 kS/s (NI 9237)"=23, "2.083 kS/s (NI 9237)"=24, "2.000 kS/s (NI 9237)"=25, "1.923 kS/s (NI 9237)"=26, "1.852 kS/s (NI 9237)"=27, "1.786 kS/s (NI 9237)"=28, "1.724 kS/s (NI 9237)"=29, "1.667 kS/s (NI 9237)"=30, "1.613 kS/s (NI 9237)"=31] ("Data Rate")
        w553 = i16 0 items=["Step", "Sine"] ("Command_p")
        w554 = i16 2 items=["Raw", "Avg.", "Avg. w. filter"] ("Strain selection_p")
        w555 = i16 0 items=["Step", "Sine"] ("Command_y")
        w556 = i16 2 items=["Raw", "Avg.", "Avg. w. filter"] ("Strain selection_y")
        w558 = fxp<+/-,25,-10> 5.851034075021744e-07  # S/F coeff_p
        w557 = fxp<+/-,25,-10> 1.0477961041033268e-06  # S/F coeff_y
        w564 = i16 0 items=["Backward", "Forward"] ("Drive mode")
        n250 = local write "Sin wave freq._y (Hz)"(fxp<+/-,32,6> 1.0 ("Sin wave freq. (Hz)")) -> ()
        n251 = local write "Sin magnitude_y"(fxp<+/-,22,7> 5.0 ("Sin magnitude")) -> ()
        n252 = local write "fy_tolorance"(fxp<+,22,6> 5.0 ("f_tolorance")) -> ()
        n253 = local write "Sin offset_y"(fxp<+/-,38,9> 0.0 ("Sin offset")) -> ()
        n254 = local write "Dyr_step"(fxp<+/-,22,7> 0.0 ("Dr")) -> ()
        n255 = local write "Kp_y"(fxp<+/-,36,9> 30.0 ("Kp")) -> ()
        n256 = local write "Kd_y"(fxp<+/-,36,9> 0.0 ("Kd")) -> ()
        n257 = local write "Kv_y"(fxp<+/-,22,8> 0.0 ("Kv")) -> ()
        n258 = local write "Bv_y"(fxp<+/-,22,8> 0.0 ("Bv")) -> ()
        n259 = local write "Ki_y"(fxp<+/-,36,9> 0.0 ("Ki")) -> ()
        n260 = local write "S/F coeff_p"(w558) -> ()
        n261 = local write "S/F coeff_y"(w557) -> ()
        n262 = local write "Data Rate"(w536) -> ()
        n263 = local write "dFy_add"(FALSE ("dF_add")) -> ()
        n264 = local write "dFp_add"(FALSE ("dFp_add")) -> ()
        n265 = local write "Sin wave freq._p (Hz)"(fxp<+/-,32,6> 1.0 ("Sin wave freq._p (Hz)")) -> ()
        n266 = local write "Sin magnitude_p"(fxp<+/-,21,6> 5.0 ("Sin magnitude_p")) -> ()
        n267 = local write "fp_tolorance"(fxp<+,22,6> 5.0 ("fp_tolorance")) -> ()
        n268 = local write "Sin offset_p"(fxp<+/-,22,7> 0.0 ("Sin offset_p")) -> ()
        n269 = local write "Dpr_step"(fxp<+/-,22,7> 0.0 ("Dpr_step")) -> ()
        n270 = local write "Kp_p"(fxp<+/-,36,9> 30.0 ("Kp_p")) -> ()
        n271 = local write "Kd_p"(fxp<+/-,36,9> 0.0 ("Kd_p")) -> ()
        n272 = local write "Kv_p"(fxp<+/-,22,8> 0.0 ("Kv_p")) -> ()
        n273 = local write "Bv_p"(fxp<+/-,22,8> 0.0 ("Bv_p")) -> ()
        n274 = local write "Ki_p"(fxp<+/-,36,9> 0.0 ("Ki_p")) -> ()
        n275 = local write "Strain selection_p"(w554) -> ()
        n276 = local write "Strain selection_y"(w556) -> ()
        n277 = local write "Command_p"(w553) -> ()
        n278 = local write "Command_y"(w555) -> ()
        n279 = local write "Drive mode"(w564) -> ()
        n280 = local write "Dp_d_M_avg_Tc (uSec)"(u32 1000 ("D_d_M_avg_Tc (uSec)")) -> ()
        n281 = local write "Dy_d_M_avg_Tc (uSec)"(1000 ("Dy_d_M_avg_Tc (uSec)")) -> ()
        n282 = local write "Belt_out_p"(fxp<+/-,7,7> 36.0 ("Belt_op")) -> ()
        n283 = local write "Belt_out_y"(fxp<+/-,7,7> 22.0 ("Belt_oy")) -> ()
        n284 = local write "Belt_in_p"(fxp<+/-,6,6> 14.0 ("Belt_mp")) -> ()
        n285 = local write "Belt_in_y"(fxp<+/-,6,6> 16.0 ("Belt_my")) -> ()
      }
    }
  }
  n286 = while "FIFO" {
    stop <- FALSE stop-if-true
    n287 = flat-sequence {
      frame #0 {
        n288 = call "Loop Timer"("Count(uSec)"=u32 1000) -> ()  [unwired: 1 out]
      }
      frame #1 {
        n289 = case shown="2" "FIFO" {
          tunnel: [w607 w623 w639] -> w591
          tunnel: [w606 w622 w638] -> w590
          tunnel: [w605 w621 w637] -> w589
          tunnel: [w604 w620 w636] -> w588
          tunnel: [w601 w619 w633] -> w586
          tunnel: [w602 w618 w634] -> w585
          tunnel: [w603 w617 w635] -> w584
          tunnel: [w599 w616 w631] -> w583
          tunnel: [w598 w615 w630] -> w582
          tunnel: [w597 w614 w629] -> w581
          tunnel: [w596 w613 w628] -> w580
          tunnel: [w595 w612 w627] -> w579
          tunnel: [w594 w611 w626] -> w578
          tunnel: [w593 w610 w625] -> w577
          tunnel: [w592 fxp<+,1,1> 0.0 ("element") w624] -> w576
          tunnel: [w600 fxp<+,1,1> 0.0 w632] -> w574
          frame 0 {
            # "Pitch"
            n290 = local read "omega_p (Mavg w. f)"() -> (w593:fxp<+/-,36,14>)
            n291 = local read "Encoder Position_p1"() -> (w607:i32)
            n292 = local read "Encoder Position_p2"() -> (w606:i32)
            n293 = local read "D_p1"() -> (w605:fxp<+/-,32,7>)
            n294 = local read "D_p2"() -> (w604:fxp<+/-,32,7>)
            n295 = local read "omega_p1 (T)"() -> (w603:fxp<+/-,36,13>)
            n296 = local read "omega_p2 (T)"() -> (w602:fxp<+/-,36,13>)
            n297 = local read "omega_p (Mavg)"() -> (w601:fxp<+/-,36,14>)
            n298 = local read "rad_p1"() -> (w600:fxp<+/-,33,20>)
            n299 = local read "rad_p2"() -> (w599:fxp<+/-,33,20>)
            n300 = local read "Force_p"() -> (w598:fxp<+/-,32,10>)
            n301 = local read "Raw Strain_p"() -> (w597:fxp<+/-,36,4>)
            n302 = local read "Strain_p (Avg8)"() -> (w596:fxp<+/-,36,4>)
            n303 = local read "Strain_p (Avg8 w. f)"() -> (w595:fxp<+/-,36,8>)
            n304 = local read "Dp_d (mm/s)"() -> (w594:fxp<+/-,36,13>)
            n305 = local read "Dp_d (Mavg)"() -> (w592:fxp<+/-,36,14>)
          }
          frame 1, Default {
            # "imp ctrl"
            n306 = local read "D_y(mm)"() -> (w623:fxp<+/-,32,7>)
            n307 = local read "Raw Strain_y"() -> (w622:fxp<+/-,36,4>)
            n308 = local read "Strain_y (Avg8)"() -> (w621:fxp<+/-,36,4>)
            n309 = local read "Strain_y (Avg8 w. f)"() -> (w620:fxp<+/-,36,8>)
            n310 = local read "Force_y"() -> (w617:fxp<+/-,32,10>)
            n311 = local read "Dy_d (T)"() -> (w618:fxp<+/-,36,13>)
            n312 = local read "Fy_dc"() -> (w619:fxp<+/-,32,10>)
            n313 = local read "D_p(mm)"() -> (w616:fxp<+/-,32,7>)
            n314 = local read "Raw Strain_p"() -> (w615:fxp<+/-,36,4>)
            n315 = local read "Strain_p (Avg8)"() -> (w614:fxp<+/-,36,4>)
            n316 = local read "Strain_p (Avg8 w. f)"() -> (w613:fxp<+/-,36,8>)
            n317 = local read "Force_p"() -> (w612:fxp<+/-,32,10>)
            n318 = local read "Dp_d (mm/s)"() -> (w611:fxp<+/-,36,13>)
            n319 = local read "Fp_dc"() -> (w610:fxp<+/-,32,10>)
          }
          frame 2 {
            # "Yaw"
            n320 = local read "omega_y (Mavg w. f.)"() -> (w625:fxp<+/-,36,14>)
            n321 = local read "Encoder Position_y1"() -> (w639:i32)
            n322 = local read "Encoder Position_y2"() -> (w638:i32)
            n323 = local read "D_y1"() -> (w637:fxp<+/-,32,7>)
            n324 = local read "D_y2"() -> (w636:fxp<+/-,32,7>)
            n325 = local read "omega_y1 (T)"() -> (w635:fxp<+/-,36,13>)
            n326 = local read "omega_y2 (T)"() -> (w634:fxp<+/-,36,13>)
            n327 = local read "omega_y (Mavg)"() -> (w633:fxp<+/-,36,14>)
            n328 = local read "rad_y1"() -> (w632:fxp<+/-,33,20>)
            n329 = local read "rad_y2"() -> (w631:fxp<+/-,33,20>)
            n330 = local read "Force_y"() -> (w630:fxp<+/-,32,10>)
            n331 = local read "Raw Strain_y"() -> (w629:fxp<+/-,36,4>)
            n332 = local read "Strain_y (Avg8)"() -> (w628:fxp<+/-,36,4>)
            n333 = local read "Strain_y (Avg8 w. f)"() -> (w627:fxp<+/-,36,8>)
            n334 = local read "Dy_d (mm/s)"() -> (w626:fxp<+/-,36,13>)
            n335 = local read "Dy_d (Mavg)"() -> (w624:fxp<+/-,36,14>)
          }
        }
        n336 = Build Array(w591, w590, w589, w588, w584, w585, w586, w574, w583, w582, w581, w580, w579, w578, w577, w576) -> (w575:fxp<+/-,64,32>[])
        n337 = xnode ("FIFO Write")("Element"=w575, "Timeout"=0) -> ()  [unwired: 1 in, 2 out]
      }
    }
  }
  n338 = while "PID force controller_y" {
    stop <- FALSE stop-if-true
    n339 = local read "Force_y"() -> (w641:fxp<+/-,32,10>)
    n340 = local read "fyt_d"() -> (w650:fxp<+/-,36,18>)
    n341 = local read "Fr_y"() -> (w642:fxp<+/-,32,10>)
    n342 = Subtract(x=w642, y=w641) -> (x-y=w640:fxp<+/-,33,11>)
    "fy_tilde" <- w640
    n343 = Absolute Value(x=w640) -> (abs(x)=w657:fxp<+,32,10>)
    n344 = local read "fyt_i"() -> (w646:fxp<+/-,36,16>)
    n345 = Multiply(x="Kp_y", y=w640) -> (x*y=w648:fxp<+/-,64,23>)
    n346 = Multiply(x="Kd_y", y=w650) -> (x*y=w649:fxp<+/-,64,27>)
    n347 = Multiply(x="Ki_y", y=w646) -> (x*y=w644:fxp<+/-,64,25>)
    n348 = Add(x=w648, y=w649) -> (x+y=w645:fxp<+/-,64,28>)
    n349 = Greater?(x=w657, y="fy_tolorance") -> (0:w655:bool)
    n350 = Add(x=w645, y=w644) -> (x+y=w643:fxp<+/-,36,16>)
    n351 = Select(t=w643, s=w655, f=fxp<+/-,51,14> 0.0) -> (s? t:f=→"Fy_PID":fxp<+/-,53,16>)
  }
  n352 = while {
    tunnel: w16 -> [w703]
    tunnel: [w677] -> w9
    shift-right: [w701] -> _
    shift-left: _ -> [w702]
    shift-right: [w697] -> _
    shift-left: _ -> [w698]
    shift-right: [w692] -> _
    shift-left: _ -> [w691]
    shift-right: [w691] -> _
    shift-left: _ -> [w690]
    shift-right: [w690] -> _
    shift-left: _ -> [w689]
    shift-right: [w689] -> _
    shift-left: _ -> [w688]
    shift-right: [w688] -> _
    shift-left: _ -> [w687]
    shift-right: [w687] -> _
    shift-left: _ -> [w686]
    shift-right: [w686] -> _
    shift-left: _ -> [w685]
    tunnel: w16 -> [w681]
    shift-right: [w674] -> _
    shift-left: _ -> [w675]
    shift-right: [w670] -> _
    shift-left: _ -> [w669]
    shift-right: [w669] -> _
    shift-left: _ -> [w668]
    shift-right: [w668] -> _
    shift-left: _ -> [w667]
    shift-right: [w667] -> _
    shift-left: _ -> [w666]
    shift-right: [w666] -> _
    shift-left: _ -> [w665]
    shift-right: [w665] -> _
    shift-left: _ -> [w664]
    shift-right: [w664] -> _
    shift-left: _ -> [w663]
    stop <- w678 stop-if-true
    w672 = fxp<+,20,2> 2.115001678466797  # Gage Factor
    n353 = xnode "FPGA I/O Node"("error in"=w703) -> ("error out"=w677:errorcluster, "Mod6/AI2"=w699:fxp<+/-,24,-4>)  [unwired: 1 in, 1 out]
    n354 = xnode "FPGA I/O Node"("error in"=w681) -> ("error out"=w679:errorcluster, "Mod6/AI3"=w673:fxp<+/-,24,-4>)  [unwired: 1 in, 1 out]
    n355 = Or(x=w677, y="Stop (Strain)") -> (x .or. y?=w680:bool)
    n356 = Select(t=w673, s="Strain gage reset_p", f=w675) -> (s? t:f=w674:fxp<+/-,24,-4>)
    n357 = Select(t=w699, s="Strain gage reset_y", f=w702) -> (s? t:f=w701:fxp<+/-,24,-4>)
    n358 = Or(x=w680, y=w679) -> (x .or. y?=w678:bool)
    n359 = Subtract(x=w673, y=w674) -> (x-y=w671:fxp<+/-,30,-3>)
    "Mod6/AI3" <- w671
    n360 = Subtract(x=w699, y=w701) -> (x-y=w700:fxp<+/-,30,-3>)
    "Mod6/AI2" <- w700
    n361 = Multiply(x=w672, y=w700) -> (x*y=w692:fxp<+/-,41,6>)
    "Raw Strain_y" <- w692
    n362 = Multiply(x=w672, y=w671) -> (x*y=w670:fxp<+/-,50,-1>)
    "Raw Strain_p" <- w670
    n363 = call "average_v2.vi"("Numeric 8"=w663, "Numeric"=w670, "Numeric 7"=w664, "Numeric 2"=w669, "Numeric 6"=w665, "Numeric 5"=w666, "Numeric 4"=w667, "Numeric 3"=w668) -> ("Mean (8pt)"=w662:fxp<+/-,32,4>)  [unwired: 1 in, 2 out]
    "Strain_p (Avg8)" <- w662
    n364 = call "average_v2.vi"("Numeric 8"=w685, "Numeric"=w692, "Numeric 7"=w686, "Numeric 2"=w691, "Numeric 6"=w687, "Numeric 5"=w688, "Numeric 4"=w689, "Numeric 3"=w690) -> ("Mean (8pt)"=w684:fxp<+/-,32,4>)  [unwired: 1 in, 2 out]
    "Strain_y (Avg8)" <- w684
    n365 = call "Tick Count"() -> ("Tick Count(uSec)"=w697:u32)
    n366 = xnode "Butterworth Filter"("input data"=w662, "scaled coefficients"="Strain_p Avg.8 coeff.") -> ("output data"=→"Strain_p (Avg8 w. f)":fxp<+/-,36,8>)  [unwired: 1 in]
    n367 = xnode "Butterworth Filter"("input data"=w684, "scaled coefficients"="Strain_y Avg8 coeff.") -> ("output data"=→"Strain_y (Avg8 w. f)":fxp<+/-,32,4>)  [unwired: 1 in]
    n368 = Subtract(x=w697, y=w698) -> (x-y=w695:fxp<+/-,32,16>)
    n369 = Divide(x=fxp<+,7,10> 1000.0, y=w695) -> (x/y=→"Loop rate (kHz)":fxp<+/-,40,27>)
  }
  n370 = for {
    N: w5 -> [_]
    tunnel: [w722] -> w4 mode=indexing
    tunnel: [w721] -> w3 mode=indexing
    tunnel: ["Dy_d_M_avg_Tc (uSec)"] -> w2
    n371 = local read "Encoder Position_y"() -> (w721:i32)
    n372 = call "Wait3"("Count(uSec)"="Dy_d_M_avg_Tc (uSec)") -> ("Tick Count(uSec)"=w722:u32)
  }
  n373 = for {
    N: w8 -> [_]
    tunnel: ["Dp_d_M_avg_Tc (uSec)"] -> w1
    tunnel: [w724] -> w7 mode=indexing
    tunnel: [w723] -> w6 mode=indexing
    n374 = local read "Encoder Position_p"() -> (w723:i32)
    n375 = call "Wait2"("Count(uSec)"="Dp_d_M_avg_Tc (uSec)") -> ("Tick Count(uSec)"=w724:u32)
  }
  n376 = while "Omega_y (Mavg)" {
    tunnel: w5 -> [w749]
    shift-right: [w747] -> _
    shift-left: w4 -> [w752]
    shift-right: [w746] -> _
    shift-left: w3 -> [w748]
    shift-right: [w741] -> _
    shift-left: _ -> [w745]
    tunnel: w2 -> [w740]
    stop <- FALSE stop-if-true
    w728 = fxp<+/-,32,0> 0.3183098859153688  # L/2/pi
    w737 = fxp<+,32,0> 0.1953125  # 800/4096
    w743 = fxp<+/-,27,3> 0.007853984832763672  # 2*pi/800
    n377 = call "Tick Count6"() -> ("Tick Count(uSec)"=w753:u32)
    n378 = Index Array(array=w752, index=0) -> (element=w751:u32)
    n379 = Index Array(array=w748, index=0) -> (element=w750:i32)
    n380 = Multiply(x=w749, y=w740) -> (x*y=w755:i32)
    n381 = Add(x=w755, y=w751) -> (x+y=w754:u32)
    n382 = Greater Or Equal?(x=w753, y=w754) -> (x >= y?=w744:bool)
    n383 = case shown="True" w744 {
      tunnel: w753 -> [_ w776]
      tunnel: w749 -> [_ w773]
      tunnel: w752 -> [w760 w775]
      tunnel: w751 -> [_ w774]
      tunnel: w750 -> [_ w770]
      tunnel: w748 -> [w759 w772]
      tunnel: [w758 w768] -> w741
      tunnel: [w760 w767] -> w747
      tunnel: [w759 w766] -> w746
      tunnel: w745 -> [w758 _]
      frame False {
      }
      frame True {
        # "count/s"
        n384 = local read "Encoder Position_y"() -> (w769:i32)
        n385 = Subtract(x=w776, y=w774) -> (x-y=w777:u32)
        n386 = Insert Into Array(array=w775, new element=w776) -> (w779:u32[])  [unwired: 1 in]
        n387 = Subtract(x=w769, y=w770) -> (x-y=w764:i32)
        n388 = Insert Into Array(array=w772, index=w773, new element=w769) -> (w780:i32[])
        n389 = To Fixed-Point(number=w777) -> (fixed-point=w763:fxp<+,32,32>)  [unwired: 1 in]
        n390 = To Fixed-Point(number=w764) -> (fixed-point=w771:fxp<+/-,32,32>)  [unwired: 1 in]
        n391 = Divide(x=w763, y=fxp<+,32,32> 1000000.0) -> (x/y=w762:fxp<+/-,64,32>)
        n392 = Delete From Array(array=w779, length=1, index=0) -> (array with subset deleted=w767:u32[])  [unwired: 1 out]
        n393 = Delete From Array(array=w780, length=1, index=0) -> (array with subset deleted=w766:i32[])  [unwired: 1 out]
        n394 = Divide(x=w771, y=w762) -> (x/y=w768:fxp<+/-,40,20>)
      }
    }
    n395 = local read "Mag. factor_p"() -> (w736:fxp<+/-,20,3>)
    n396 = local read "Mag. encoder_y"() -> (w739:bool)
    n397 = local read "Belt_in_y"() -> (w730:fxp<+/-,6,6>)
    n398 = Multiply(x=w743, y=w741) -> (x*y=w733:fxp<+/-,64,23>)
    n399 = Divide(x=w737, y=w736) -> (x/y=w735:fxp<+/-,32,1>)
    n400 = local read "Belt_out_y"() -> (w731:fxp<+/-,7,7>)
    n401 = Select(t=w735, s=w739, f=fxp<+/-,2,2> 1.0) -> (s? t:f=w734:fxp<+/-,33,2>)
    n402 = Multiply(x=w728, y=w730) -> (x*y=w729:fxp<+/-,38,6>)
    n403 = Multiply(x=w734, y=w733) -> (x*y=w732:fxp<+/-,64,25>)
    "omega_y (Mavg)" <- w732
    n404 = Divide(x=w729, y=w731) -> (x/y=w727:fxp<+/-,45,6>)
    n405 = Multiply(x=w727, y=w732) -> (x*y=→"Dy_d (Mavg)":fxp<+/-,64,30>)
  }
  n406 = while "Omega_p (Mavg)" {
    tunnel: w8 -> [w806]
    shift-right: [w804] -> _
    shift-left: w7 -> [w809]
    shift-right: [w803] -> _
    shift-left: w6 -> [w805]
    shift-right: [w802] -> _
    shift-left: _ -> [w801]
    tunnel: w1 -> [w799]
    stop <- FALSE stop-if-true
    w788 = fxp<+/-,27,3> 0.007853984832763672  # 2*pi/800
    w790 = fxp<+,32,0> 0.1953125  # 800/4096
    w787 = fxp<+/-,32,0> 0.3183098859153688  # L/2/pi
    n407 = call "Tick Count5"() -> ("Tick Count(uSec)"=w810:u32)
    n408 = Index Array(array=w809, index=0) -> (element=w808:u32)
    n409 = Index Array(array=w805, index=0) -> (element=w807:i32)
    n410 = Multiply(x=w806, y=w799) -> (x*y=w812:i32)
    n411 = Add(x=w812, y=w808) -> (x+y=w811:u32)
    n412 = Greater Or Equal?(x=w810, y=w811) -> (x >= y?=w800:bool)
    n413 = case shown="True" w800 {
      tunnel: w810 -> [_ w833]
      tunnel: w806 -> [_ w830]
      tunnel: w809 -> [w817 w832]
      tunnel: w808 -> [_ w831]
      tunnel: w807 -> [_ w827]
      tunnel: w805 -> [w816 w829]
      tunnel: [w815 w825] -> w802
      tunnel: [w817 w824] -> w804
      tunnel: [w816 w823] -> w803
      tunnel: w801 -> [w815 _]
      frame False {
      }
      frame True {
        n414 = local read "Encoder Position_p"() -> (w826:i32)
        n415 = Subtract(x=w833, y=w831) -> (x-y=w834:u32)
        n416 = Subtract(x=w826, y=w827) -> (x-y=w818:i32)
        n417 = Insert Into Array(array=w832, new element=w833) -> (w836:u32[])  [unwired: 1 in]
        n418 = Insert Into Array(array=w829, index=w830, new element=w826) -> (w837:i32[])
        n419 = To Fixed-Point(number=w834) -> (fixed-point=w820:fxp<+,32,32>)  [unwired: 1 in]
        n420 = To Fixed-Point(number=w818) -> (fixed-point=w828:fxp<+/-,32,32>)  [unwired: 1 in]
        n421 = Delete From Array(array=w836, length=1, index=0) -> (array with subset deleted=w824:u32[])  [unwired: 1 out]
        n422 = Delete From Array(array=w837, length=1, index=0) -> (array with subset deleted=w823:i32[])  [unwired: 1 out]
        n423 = Divide(x=w820, y=fxp<+,32,32> 1000000.0) -> (x/y=w821:fxp<+/-,64,32>)
        n424 = Divide(x=w828, y=w821) -> (x/y=w825:fxp<+/-,40,20>)
      }
    }
    n425 = local read "Mag. factor_p"() -> (w791:fxp<+/-,20,3>)
    n426 = local read "Mag. encoder_p"() -> (w798:bool)
    n427 = local read "Belt_in_p"() -> (w795:fxp<+/-,6,6>)
    n428 = Divide(x=w790, y=w791) -> (x/y=w789:fxp<+/-,32,1>)
    n429 = local read "Belt_out_p"() -> (w794:fxp<+/-,7,7>)
    n430 = Multiply(x=w788, y=w802) -> (x*y=w796:fxp<+/-,64,23>)
    n431 = Select(t=w789, s=w798, f=fxp<+/-,2,2> 1.0) -> (s? t:f=w783:fxp<+/-,33,2>)
    n432 = Multiply(x=w787, y=w795) -> (x*y=w793:fxp<+/-,38,6>)
    n433 = Multiply(x=w783, y=w796) -> (x*y=w786:fxp<+/-,64,25>)
    "omega_p (Mavg)" <- w786
    n434 = Divide(x=w793, y=w794) -> (x/y=w785:fxp<+/-,45,6>)
    n435 = Multiply(x=w785, y=w786) -> (x*y=→"Dp_d (Mavg)":fxp<+/-,64,30>)
  }
  n436 = while "Quadrature drive_p" {
    stop <- FALSE stop-if-true
    n437 = local read "dFp_PID"() -> (w841:fxp<+/-,36,18>)
    n438 = local read "omega_p (rad/s)"() -> (w847:fxp<+/-,36,13>)
    n439 = local read "Fp_PID"() -> (w842:fxp<+/-,36,16>)
    n440 = Select(t=w841, s="dFp_add", f=fxp<+,1,1> 0.0) -> (s? t:f=w845:fxp<+/-,36,18>)
    n441 = call "Oriental_step_motor_PKP225.vi"("F_Threshold"=fxp<+,12,12> 10.0, "dFmr"=w845, "omega"=w847, "Fmr"=w842) -> ("vq_F"=→"vq_p_F":fxp<+/-,20,5>, "vd_F"=→"vd_p_F":fxp<+/-,20,5>)  [unwired: 6 in]
  }
  n442 = while "PID force controller_p" {
    shift-right: [w854] -> _
    shift-left: _ -> [w853]
    stop <- FALSE stop-if-true
    n443 = local read "Force_p"() -> (w866:fxp<+/-,32,10>)
    n444 = local read "fpt_d"() -> (w862:fxp<+/-,36,18>)
    n445 = local read "Fr_p"() -> (w867:fxp<+/-,32,10>)
    n446 = Subtract(x=w867, y=w866) -> (x-y=w864:fxp<+/-,33,11>)
    "fp_tilde" <- w864
    n447 = local read "fpt_i"() -> (w858:fxp<+/-,34,18>)
    n448 = Multiply(x="Kp_p", y=w864) -> (x*y=w860:fxp<+/-,64,23>)
    n449 = Multiply(x="Kd_p", y=w862) -> (x*y=w861:fxp<+/-,64,27>)
    n450 = Absolute Value(x=w864) -> (abs(x)=w873:fxp<+,32,10>)
    n451 = Add(x=w860, y=w861) -> (x+y=w856:fxp<+/-,64,28>)
    n452 = Multiply(x="Ki_p", y=w858) -> (x*y=w857:fxp<+/-,64,27>)
    n453 = call "Tick Count7"() -> ("Tick Count(uSec)"=w854:u32)
    n454 = Add(x=w856, y=w857) -> (x+y=w855:fxp<+/-,36,16>)
    n455 = Greater?(x=w873, y="fp_tolorance") -> (0:w870:bool)
    n456 = Subtract(x=w854, y=w853) -> (x-y=w852:u32)
    n457 = Divide(x=u32 1000, y=w852) -> (x/y=→"PID (kHz)":fxp<+/-,20,7>)
    n458 = Select(t=w855, s=w870, f=fxp<+,1,1> 0.0) -> (s? t:f=→"Fp_PID":fxp<+/-,36,16>)
  }
  n459 = while "PD position controller_p" {
    stop <- FALSE stop-if-true
    n460 = local read "Drive mode"() -> (w876:i16)
    n461 = case shown="1" w876 {
      tunnel: [fxp<+/-,62,19> 0.0 w879] -> w875
      frame 0, Default {
        # "Backward"
      }
      frame 1 {
        # "Forward"
        n462 = local read "D_p(mm)"() -> (w886:fxp<+/-,32,7>)
        n463 = local read "Dp_error_d"() -> (w878:fxp<+/-,33,8>)
        n464 = local read "Dpr_for"() -> (w885:fxp<+/-,22,7>)
        n465 = Subtract(x=w885, y=w886) -> (x-y=w884:fxp<+/-,24,8>)
        "Dp_error" <- w884
        n466 = Multiply(x=w884, y="Kv_p") -> (x*y=w881:fxp<+/-,34,16>)
        n467 = Multiply(x=w878, y="Bv_p") -> (x*y=w880:fxp<+/-,55,16>)
        n468 = Add(x=w881, y=w880) -> (x+y=w879:fxp<+/-,56,17>)
      }
    }
    "Fr_p" <- w875
  }
  n469 = while "All switch" {
    stop <- FALSE stop-if-true
    n470 = case shown="True" "Encoder reset" {
      frame False {
        n471 = local write "Encoder reset_p"(FALSE ("Encoder reset_p")) -> ()
        n472 = local write "Encoder reset_y"(FALSE ("Encoder reset_y")) -> ()
      }
      frame True {
        n473 = flat-sequence {
          frame #0 {
            n474 = local write "Encoder reset_p"(TRUE ("Encoder reset_p")) -> ()
          }
          frame #1 {
            n475 = local write "Encoder reset_y"(TRUE ("Encoder reset_y")) -> ()
            n476 = local write "Encoder reset_p"(FALSE ("Encoder reset_p")) -> ()
          }
          frame #2 {
            n477 = local write "Encoder reset_y"(FALSE ("Encoder reset_y")) -> ()
          }
        }
      }
    }
  }
  n478 = while "Derivative" {
    stop <- FALSE stop-if-true
    n479 = local read "Dpr_sin_dd"() -> (w903:fxp<+/-,35,20>)
    n480 = local read "Stop motor_y"() -> (w909:bool)
    n481 = local read "Dyr_sin_dd"() -> (w911:fxp<+/-,35,20>)
    n482 = local read "Dpr_sin_d"() -> (w905:fxp<+/-,33,15>)
    n483 = local read "Stop motor_p"() -> (w901:bool)
    n484 = local read "Dyr_sin_d"() -> (w914:fxp<+/-,33,15>)
    n485 = local read "Dp_error"() -> (w906:fxp<+/-,22,7>)
    n486 = local read "Dy_error"() -> (w915:fxp<+/-,22,7>)
    n487 = local read "Dp_dd"() -> (w904:fxp<+/-,36,25>)
    n488 = local read "Dy_dd"() -> (w912:fxp<+/-,36,25>)
    n489 = Subtract(x=w914, y=w915) -> (x-y=w913:fxp<+/-,34,16>)
    n490 = Subtract(x=w911, y=w912) -> (x-y=w910:fxp<+/-,41,26>)
    n491 = Subtract(x=w905, y=w906) -> (x-y=w898:fxp<+/-,34,16>)
    n492 = Subtract(x=w903, y=w904) -> (x-y=w902:fxp<+/-,41,26>)
    n493 = Select(t=fxp<+,1,1> 0.0, s=w909, f=w913) -> (s? t:f=→"Dy_error_d":fxp<+/-,34,16>)
    n494 = Select(t=fxp<+/-,64,49> 0.0, s=w909, f=w910) -> (s? t:f=→"Dy_error_dd":fxp<+/-,64,49>)
    n495 = Select(t=fxp<+,1,1> 0.0, s=w901, f=w898) -> (s? t:f=→"Dp_error_d":fxp<+/-,34,16>)
    n496 = Select(t=fxp<+/-,41,26> 0.0, s=w901, f=w902) -> (s? t:f=→"Dp_error_dd":fxp<+/-,41,26>)
  }
  n497 = while "ft_d" {
    stop <- FALSE stop-if-true
    n498 = local read "Dy_error_dd"() -> (w933:fxp<+/-,36,16>)
    n499 = local read "Dp_error_dd"() -> (w924:fxp<+/-,36,16>)
    n500 = local read "Dy_error_d"() -> (w935:fxp<+/-,33,8>)
    n501 = local read "Dp_error_d"() -> (w926:fxp<+/-,33,8>)
    n502 = local read "Kv_p"() -> (w927:fxp<+/-,22,8>)
    n503 = local read "Bv_p"() -> (w925:fxp<+/-,22,8>)
    n504 = local read "Kv_y"() -> (w936:fxp<+/-,22,8>)
    n505 = local read "Bv_y"() -> (w934:fxp<+/-,22,8>)
    n506 = local read "Force_y"() -> (w929:fxp<+/-,32,10>)
    n507 = Multiply(x=w935, y=w936) -> (x*y=w931:fxp<+/-,55,16>)
    n508 = Multiply(x=w933, y=w934) -> (x*y=w932:fxp<+/-,58,24>)
    n509 = Multiply(x=w926, y=w927) -> (x*y=w922:fxp<+/-,55,16>)
    n510 = Multiply(x=w924, y=w925) -> (x*y=w923:fxp<+/-,58,24>)
    n511 = local read "Force_p"() -> (w920:fxp<+/-,32,10>)
    n512 = Add(x=w931, y=w932) -> (x+y=w930:fxp<+/-,63,24>)
    n513 = Add(x=w922, y=w923) -> (x+y=w921:fxp<+/-,63,24>)
    n514 = Subtract(x=w930, y=w929) -> (x-y=→"fyt_d":fxp<+/-,63,24>)
    n515 = Subtract(x=w921, y=w920) -> (x-y=→"fpt_d":fxp<+/-,63,24>)
  }
  n516 = while "Encoder_y" {
    shift-right: [w975] -> _
    shift-left: _ -> [w967]
    shift-right: [w974] -> _
    shift-left: _ -> [w966]
    shift-right: [w965] -> _
    shift-left: _ -> [w963]
    shift-right: [w971] -> _
    shift-left: _ -> [w968]
    shift-right: [w970] -> _
    shift-left: _ -> [w969]
    shift-right: [w964] -> _
    shift-left: _ -> [w962]
    stop <- FALSE stop-if-true
    w952 = fxp<+/-,16,1> 0.0244140625  # 2*50/4096
    w957 = fxp<+/-,20,-5> 0.00048828125  # L/4096
    w960 = fxp<+/-,20,-5> 0.002499997615814209  # L/800
    w942 = fxp<+/-,16,1> 0.125  # 2*50/800
    n517 = xnode "FPGA I/O Node"() -> ("Mod7/DIO2"=w976:bool, "Mod7/DIO3"=w977:bool)  [unwired: 2 in, 2 out]
    n518 = xnode "FPGA I/O Node"() -> ("Mod7/DIO6"=w973:bool, "Mod7/DIO7"=w972:bool)  [unwired: 2 in, 2 out]
    n519 = local read "Encoder reset_y"() -> (w947:bool)
    n520 = call "encoder_sub.vi"("A_pre"=w967, "B_pre"=w966, "Encoder Position_pre"=w963, "A input"=w976, "Encoder Position Reset"="Encoder reset_y", "B input"=w977) -> ("A"=w975:bool, "B"=w974:bool, "Encoder Position (Counts)"=w965:i32)  [unwired: 19 in]
    "Encoder Position_y1" <- w965
    n521 = call "encoder_sub.vi"("A_pre"=w968, "B_pre"=w969, "Encoder Position_pre"=w962, "A input"=w973, "Encoder Position Reset"=w947, "B input"=w972) -> ("A"=w971:bool, "B"=w970:bool, "Encoder Position (Counts)"=w964:i32)  [unwired: 19 in]
    "Encoder Position_y2" <- w964
    n522 = local read "Belt_in_y"() -> (w955:fxp<+/-,6,6>)
    n523 = local read "Belt_in_y"() -> (w959:fxp<+/-,6,6>)
    n524 = local read "Belt_out_y"() -> (w953:fxp<+/-,7,7>)
    n525 = Divide(x=w957, y="Mag. factor_y") -> (x/y=w956:fxp<+/-,41,13>)
    n526 = local read "Belt_out_y"() -> (w958:fxp<+/-,7,7>)
    n527 = To Fixed-Point(number=w964) -> (fixed-point=w939:fxp<+/-,32,32>)  [unwired: 1 in]
    n528 = local read "Mag. factor_y"() -> (w951:fxp<+/-,20,3>)
    n529 = To Fixed-Point(number=w965) -> (fixed-point=w943:fxp<+/-,32,32>)  [unwired: 1 in]
    n530 = Multiply(x=w956, y=w955) -> (x*y=w954:fxp<+/-,46,18>)
    n531 = Multiply(x=w960, y=w959) -> (x*y=w961:fxp<+/-,26,1>)
    n532 = Divide(x=w954, y=w953) -> (x/y=w941:fxp<+/-,53,18>)
    n533 = Divide(x=w961, y=w958) -> (x/y=w945:fxp<+/-,33,1>)
    n534 = Divide(x=w952, y=w951) -> (x/y=w938:fxp<+/-,32,1>)
    n535 = Multiply(x=w941, y=w939) -> (x*y=→"D_y2":fxp<+/-,37,7>)
    n536 = Multiply(x=w943, y=w942) -> (x*y=→"rad_y1":fxp<+/-,33,20>)
    n537 = Multiply(x=w945, y=w943) -> (x*y=→"D_y1":fxp<+/-,32,7>)
    n538 = Multiply(x=w939, y=w938) -> (x*y=→"rad_y2":fxp<+/-,33,20>)
  }
  n539 = while "Omega_y(T method)" {
    shift-right: [w1004] -> _
    shift-left: _ -> [w1005]
    shift-right: [w981] -> _
    shift-left: _ -> [w1007]
    shift-right: [w1009] -> _
    shift-left: _ -> [w1010]
    shift-right: [w997] -> _
    shift-left: _ -> [w995]
    shift-right: [w990] -> _
    shift-left: _ -> [w996]
    shift-right: [w993] -> _
    shift-left: _ -> [w994]
    stop <- FALSE stop-if-true
    w988 = fxp<+/-,32,0> 0.3183098859153688  # L/2/pi
    w999 = fxp<+,32,0> 0.1953125  # 800/4096
    w1003 = fxp<+/-,32,0> 0.3183098859153688  # L/2/pi
    n540 = local read "Encoder Position_y1"() -> (w1004:i32)
    n541 = call "Tick Count2"() -> ("Tick Count(Ticks)"=w991:u32)
    n542 = local read "Encoder Position_y2"() -> (w997:i32)
    n543 = local read "Mag. factor_y"() -> (w998:fxp<+/-,20,3>)
    n544 = call "omega_sub_Encoder_800ppr.vi"("mt0"="mt0_omega_y", "omega_pre"=w1007, "ticks_m_pre"=w1010, "ticks"=w991, "count_pre"=w1005, "count"=w1004) -> ("ticks_m"=w1009:u32, "mt"=→"mt_omega_y1":u32, "omega"=w981:fxp<+/-,36,13>)  [unwired: 3 in]
    "omega_y1 (T)" <- w981
    n545 = call "omega_sub_Encoder_800ppr.vi"("omega_pre"=w996, "ticks_m_pre"=w994, "ticks"=w991, "count_pre"=w995, "count"=w997) -> ("ticks_m"=w993:u32, "mt"=→"mt_omega_y2":u32, "omega"=w990:fxp<+/-,36,13>)  [unwired: 4 in]
    n546 = local read "Belt_in_y"() -> (w987:fxp<+/-,6,6>)
    n547 = local read "Belt_out_y"() -> (w985:fxp<+/-,7,7>)
    n548 = Divide(x=w999, y=w998) -> (x/y=w989:fxp<+/-,32,1>)
    n549 = Multiply(x=w1003, y="Belt_in_y") -> (x*y=w1001:fxp<+/-,38,6>)
    n550 = Multiply(x=w988, y=w987) -> (x*y=w986:fxp<+/-,38,6>)
    n551 = Divide(x=w986, y=w985) -> (x/y=w979:fxp<+/-,45,6>)
    n552 = Divide(x=w1001, y="Belt_out_y") -> (x/y=w982:fxp<+/-,20,1>)
    n553 = Multiply(x=w990, y=w989) -> (x*y=w978:fxp<+/-,36,13>)
    "omega_y2 (T)" <- w978
    n554 = Multiply(x=w982, y=w981) -> (x*y=→"Dy1_d (T)":fxp<+/-,36,13>)
    n555 = Multiply(x=w979, y=w978) -> (x*y=→"Dy2_d (T)":fxp<+/-,36,13>)
  }
  n556 = xnode "FPGA I/O Node"("error in"=w9, "Mod6/Stop"=TRUE) -> ()  [unwired: 1 in, 2 out]
  n557 = while {
    stop <- FALSE stop-if-true
    n558 = case shown="True" "Set 3" {
      frame False {
      }
      frame True {
        n559 = local write "fp_tolorance"(fxp<+,22,6> 3.0 ("fp_tolorance")) -> ()
        n560 = local write "Kp_p"(fxp<+/-,36,9> 100.0 ("Kp_p")) -> ()
      }
    }
    n561 = case shown="True" "Set 2" {
      frame False {
      }
      frame True {
        n562 = local write "fp_tolorance"(fxp<+,22,6> 1.5 ("fp_tolorance")) -> ()
        n563 = local write "Kp_p"(fxp<+/-,36,9> 50.0 ("Kp_p")) -> ()
      }
    }
    n564 = case shown="True" "Set 1" {
      frame False {
      }
      frame True {
        n565 = local write "fp_tolorance"(fxp<+,22,6> 3.0 ("fp_tolorance")) -> ()
        n566 = local write "Kp_p"(fxp<+/-,36,9> 50.0 ("Kp_p")) -> ()
      }
    }
    n567 = case shown="True" "Set 5" {
      frame False {
      }
      frame True {
        n568 = local write "fp_tolorance"(fxp<+,22,6> 3.0 ("fp_tolorance")) -> ()
        n569 = local write "Kp_p"(fxp<+/-,36,9> 150.0 ("Kp_p")) -> ()
      }
    }
    n570 = case shown="True" "Set 6" {
      frame False {
      }
      frame True {
        n571 = local write "fp_tolorance"(fxp<+,22,6> 1.5 ("fp_tolorance")) -> ()
        n572 = local write "Kp_p"(fxp<+/-,36,9> 150.0 ("Kp_p")) -> ()
      }
    }
    n573 = case shown="True" "Set 4" {
      frame False {
      }
      frame True {
        n574 = local write "fp_tolorance"(fxp<+,22,6> 1.5 ("fp_tolorance")) -> ()
        n575 = local write "Kp_p"(fxp<+/-,36,9> 100.0 ("Kp_p")) -> ()
      }
    }
  }
  n576 = while {
    stop <- FALSE stop-if-true
    n577 = local read "omega_y (Mavg)"() -> (w1038:fxp<+/-,36,14>)
    n578 = local read "omega_p (Mavg)"() -> (w1042:fxp<+/-,36,14>)
    n579 = local read "Dp_d (Mavg)"() -> (w1034:fxp<+/-,36,14>)
    n580 = local read "Dy_d (Mavg)"() -> (w1035:fxp<+/-,36,14>)
    n581 = xnode "Butterworth Filter"("input data"=w1038, "scaled coefficients"="omega_y(Mavg) coeff.") -> ("output data"=→"omega_y (Mavg w. f.)":fxp<+/-,36,18>)  [unwired: 1 in]
    n582 = xnode "Butterworth Filter"("input data"=w1042, "scaled coefficients"="omega_P(Mavg) coeff.") -> ("output data"=→"omega_p (Mavg w. f)":fxp<+/-,36,18>)  [unwired: 1 in]
    n583 = xnode "Butterworth Filter"("input data"=w1035, "scaled coefficients"="Dy_d (Mavg) coeff.") -> ("output data"=→"Dy_d (Mavg w. f.)":fxp<+/-,36,18>)  [unwired: 1 in]
    n584 = xnode "Butterworth Filter"("input data"=w1034, "scaled coefficients"="Dp_d (Mavg) coeff.") -> ("output data"=→"Dp_d (Mavg w. f.)":fxp<+/-,36,18>)  [unwired: 1 in]
  }
